vi "WT330.vi"(7 "simulazione":bool, 8 "error in (no error)":errorcluster, 11 "Queue Name":string="WT330_Q") -> (0 "error out":errorcluster, 2 "Stopped":bool)   [LabVIEW 2019]
uses:
  TypeDef/MISURE WT.ctl
  TypeDef/DEVICE NAME.ctl
  <vilib>/Utility/file.llb/Read From Spreadsheet File (string).vi
  <instrlib>/Yokogawa WT300 Series/Public/Data/Read Measurement (Normal).vi
  Globals.vi
  Global_All_Data.vi
  <instrlib>/Yokogawa WT300 Series/Yokogawa WT300 Series.lvlib
  <instrlib>/Yokogawa WT200 Series/Yokogawa WT200 Series.lvlib
panel:
  out "error out 5":errorcluster
  out "error out 4":errorcluster
  in  "DIRETTO WT":bool
  out "error out 3":errorcluster
  in  "CT Ratio (1.000)":dbl=0.2 format="%#_13g"
  in  "write buffer":string=":INP:CURR:AUTO OFF;:INP:CURR:RANG EXT,1.0;"
  in  "LEM GENERICO":bool
  in  "Number of Item (15)":i32=39
  in  "rms mode":bool
  in  "dc mode":bool
  in  "IRMS 3":dbl
  out "error out 2":errorcluster
  in  "LEM 1000":bool
  in  "LEM 300":bool
  out "Numeric":i32
  in  "Measurement 2":dbl[](array[numeric])=[400.0, 25.0, 2409.0, 3031.0, 7.7, 0.8, 120.0, 50.0, 50.0, -1.0, 400.0, 25.0, 2409.0, 3031.0, 7.7, 0.8, 120.0, 50.0, 50.0, -1.0, 400.0, 25.0, 3030.0, 2400.0, 6.0, 0.8, 120.0, 50.0, 50.0, -1.0, 400.0, 25.0, 10104.0, 8009.0, 23.0, 0.8, 120.0, 50.0, 50.0]
  out "MISURE WT":T1
  out "WT330 Configuration":string[][](array[string])
  out "Function":string[](array[string])=["U,1\n", "I,1\n", "P,1\n", "S,1\n", "Q,1\n", "LAMB,1\n", "PHI,1\n", "FU,1\n", "FI,1\n", "NONE\n", "U,2\n", "I,2\n", "P,2\n", "S,2\n", "Q,2\n", "LAMB,2\n", "PHI,2\n", "FU,2\n", "FI,2\n", "NONE\n", "U,3\n", "I,3\n", "P,3\n", "S,3\n", "Q,3\n", "LAMB,3\n", "PHI,3\n", "FU,3\n", "FI,3\n", "NONE\n", "U,SIGM\n", "I,SIGM\n", "P,SIGM\n", "S,SIGM\n", "Q,SIGM\n", "LAMB,SIGM\n", "PHI,SIGM\n", "FU,SIGM\n", "FI,SIGM\n"]
  out "Measurement":dbl[](array[numeric])
  out "VISA resource name":refnum<visa-resource-name>
  out "STATO":string
  out "LOOP TIME (ms)":u32
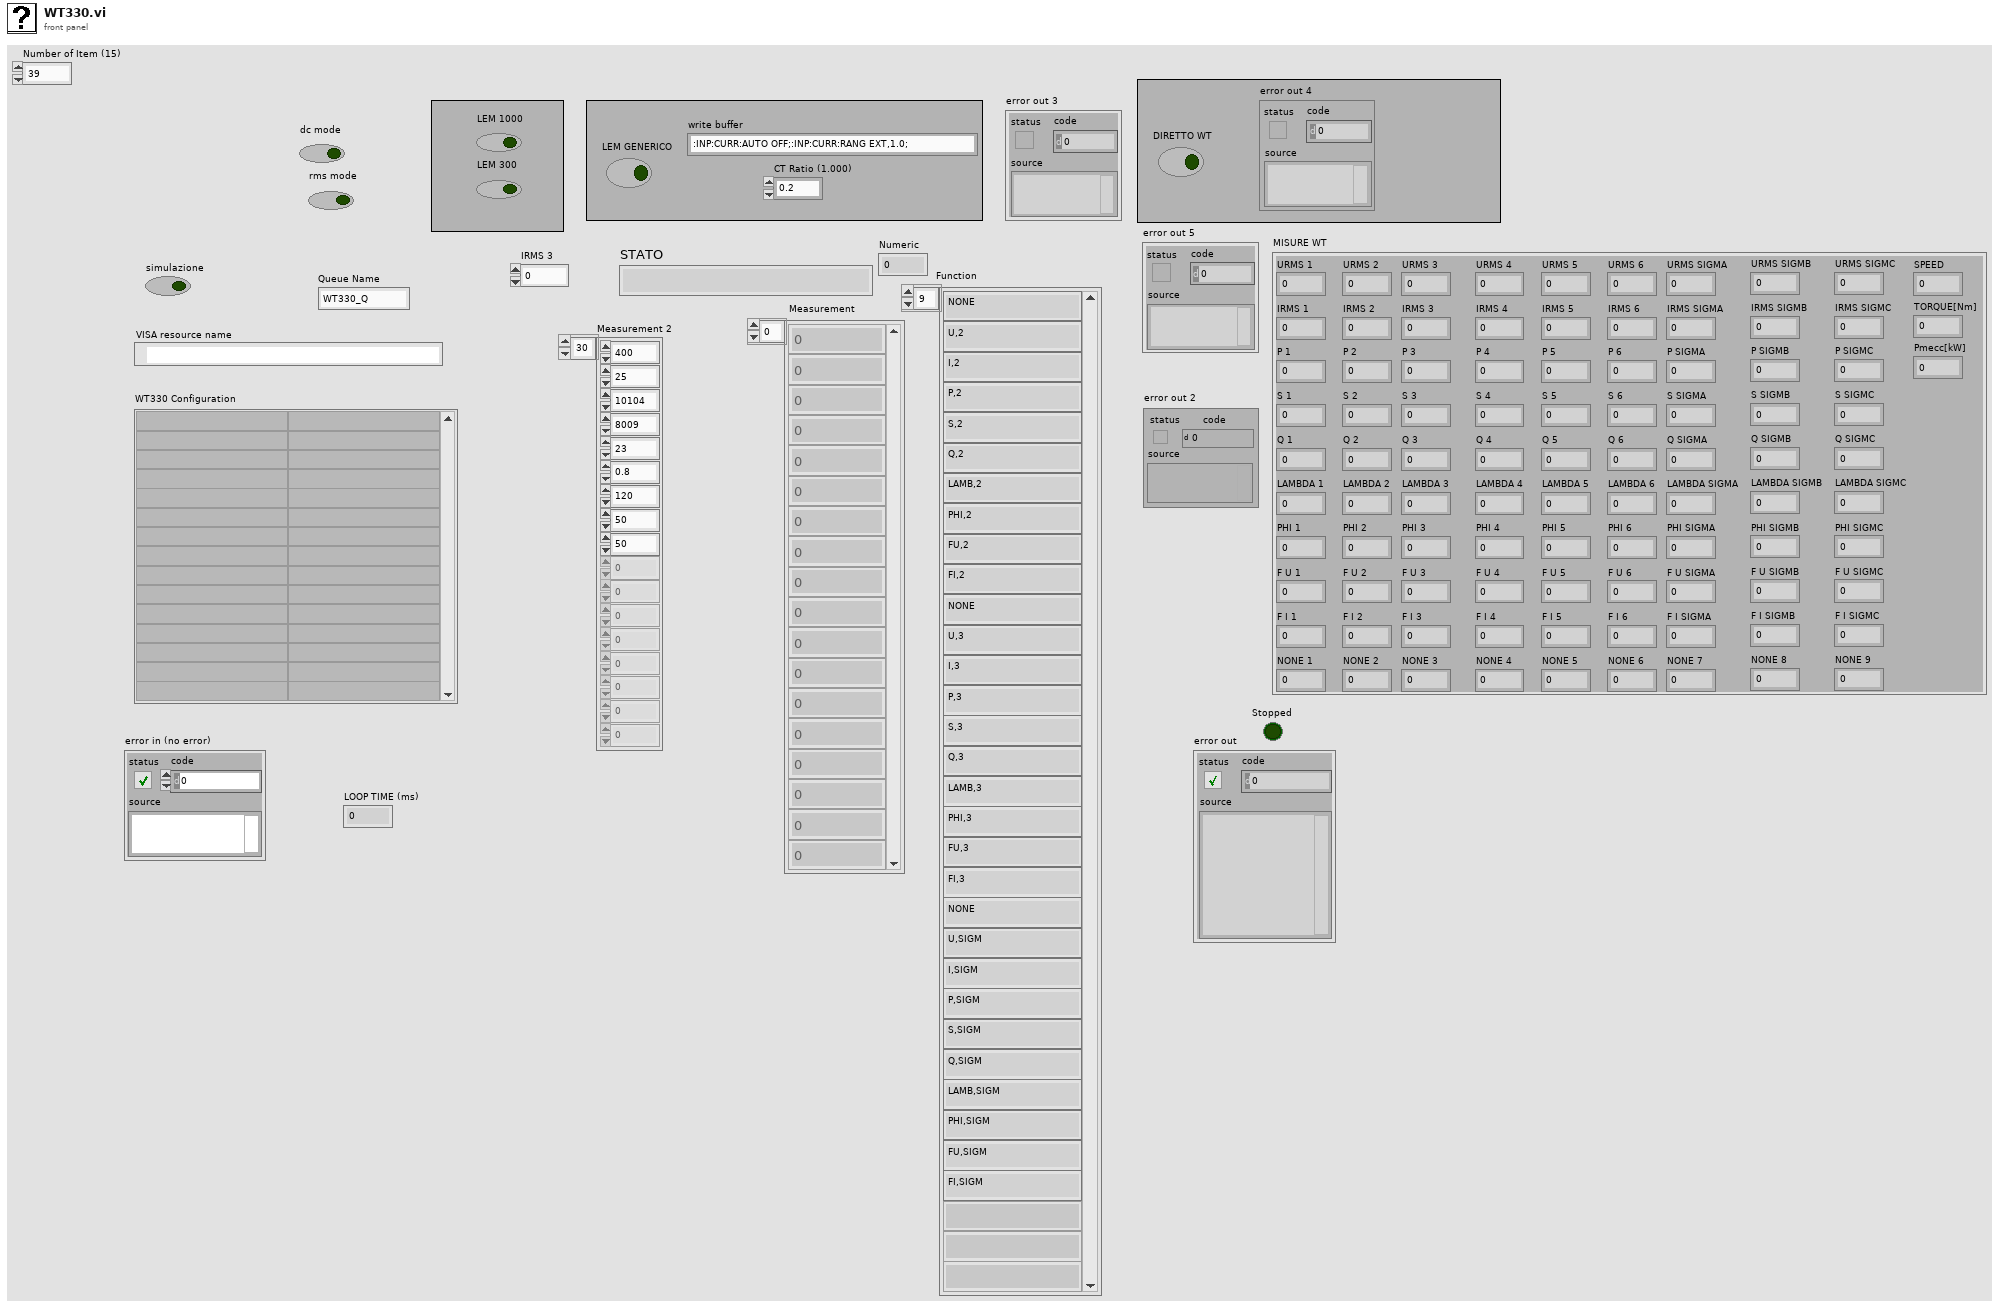
[diagram p1: front panel]
types:
  T1 = typedef "MISURE WT.ctl" = cluster{"URMS 1":dbl, "IRMS 1":dbl, "P 1":dbl, "S 1":dbl, "Q 1":dbl, "LAMBDA 1":dbl, "PHI 1":dbl, "F U 1":dbl, "F I 1":dbl, "NONE 1":dbl, "URMS 2":dbl, "IRMS 2":dbl, "P 2":dbl, "S 2":dbl, "Q 2":dbl, "LAMBDA 2":dbl, "PHI 2":dbl, "F U 2":dbl, "F I 2":dbl, "NONE 2":dbl, "URMS 3":dbl, "IRMS 3":dbl, "P 3":dbl, "S 3":dbl, "Q 3":dbl, "LAMBDA 3":dbl, "PHI 3":dbl, "F U 3":dbl, "F I 3":dbl, "NONE 3":dbl, "URMS 4":dbl, "IRMS 4":dbl, "P 4":dbl, "S 4":dbl, "Q 4":dbl, "LAMBDA 4":dbl, "PHI 4":dbl, "F U 4":dbl, "F I 4":dbl, "NONE 4":dbl, "URMS 5":dbl, "IRMS 5":dbl, "P 5":dbl, "S 5":dbl, "Q 5":dbl, "LAMBDA 5":dbl, "PHI 5":dbl, "F U 5":dbl, "F I 5":dbl, "NONE 5":dbl, "URMS 6":dbl, "IRMS 6":dbl, "P 6":dbl, "S 6":dbl, "Q 6":dbl, "LAMBDA 6":dbl, "PHI 6":dbl, "F U 6":dbl, "F I 6":dbl, "NONE 6":dbl, "URMS SIGMA":dbl, "IRMS SIGMA":dbl, "P SIGMA":dbl, "S SIGMA":dbl, "Q SIGMA":dbl, "LAMBDA SIGMA":dbl, "PHI SIGMA":dbl, "F U SIGMA":dbl, "F I SIGMA":dbl, "NONE 7":dbl, "URMS SIGMB":dbl, "IRMS SIGMB":dbl, "P SIGMB":dbl, "S SIGMB":dbl, "Q SIGMB":dbl, "LAMBDA SIGMB":dbl, "PHI SIGMB":dbl, "F U SIGMB":dbl, "F I SIGMB":dbl, "NONE 8":dbl, "URMS SIGMC":dbl, "IRMS SIGMC":dbl, "P SIGMC":dbl, "S SIGMC":dbl, "Q SIGMC":dbl, "LAMBDA SIGMC":dbl, "PHI SIGMC":dbl, "F U SIGMC":dbl, "F I SIGMC":dbl, "NONE 9":dbl, "SPEED":dbl, "TORQUE[Nm]":dbl, "Pmecc[kW]":dbl}
  T2 = typedef "DEVICE NAME.ctl" = enum16{"WATTMETRO", "APLUS", "PLC BANCO 1", "PLC RACK", "PLC BANCO 2", "PS", "NI cDAQ", "RESISTOMAT"}
  T3 = cluster{"Array of elements":cluster{"String":string, "variant":variant}[], "Single element":cluster{"String":string, "variant":variant}, "enque at\nopposite end (F)":bool, "no replications (F)":bool}
  T4 = cluster{"Measure Value[0]":dbl, "Measure Value[1]":dbl, "Measure Value[2]":dbl, "Measure Value[3]":dbl, "Measure Value[4]":dbl, "Measure Value[5]":dbl, "Measure Value[6]":dbl, "Measure Value[7]":dbl, "Measure Value[8]":dbl, "Measure Value[9]":dbl, "Measure Value[10]":dbl, "Measure Value[11]":dbl, "Measure Value[12]":dbl, "Measure Value[13]":dbl, "Measure Value[14]":dbl, "Measure Value[15]":dbl, "Measure Value[16]":dbl, "Measure Value[17]":dbl, "Measure Value[18]":dbl, "Measure Value[19]":dbl, "Measure Value[20]":dbl, "Measure Value[21]":dbl, "Measure Value[22]":dbl, "Measure Value[23]":dbl, "Measure Value[24]":dbl, "Measure Value[25]":dbl, "Measure Value[26]":dbl, "Measure Value[27]":dbl, "Measure Value[28]":dbl, "Measure Value[29]":dbl, "Measure Value[30]":dbl, "Measure Value[31]":dbl, "Measure Value[32]":dbl, "Measure Value[33]":dbl, "Measure Value[34]":dbl, "Measure Value[35]":dbl, "Measure Value[36]":dbl, "Measure Value[37]":dbl, "Measure Value[38]":dbl, "Measure Value[39]":dbl, "Measure Value[40]":dbl, "Measure Value[41]":dbl, "Measure Value[42]":dbl, "Measure Value[43]":dbl, "Measure Value[44]":dbl, "Measure Value[45]":dbl, "Measure Value[46]":dbl, "Measure Value[47]":dbl, "Measure Value[48]":dbl, "Measure Value[49]":dbl, "Measure Value[50]":dbl, "Measure Value[51]":dbl, "Measure Value[52]":dbl, "Measure Value[53]":dbl, "Measure Value[54]":dbl, "Measure Value[55]":dbl, "Measure Value[56]":dbl, "Measure Value[57]":dbl, "Measure Value[58]":dbl, "Measure Value[59]":dbl, "Measure Value[60]":dbl, "Measure Value[61]":dbl, "Measure Value[62]":dbl, "Measure Value[63]":dbl, "Measure Value[64]":dbl, "Measure Value[65]":dbl, "Measure Value[66]":dbl, "Measure Value[67]":dbl, "Measure Value[68]":dbl, "Measure Value[69]":dbl, "Measure Value[70]":dbl, "Measure Value[71]":dbl, "Measure Value[72]":dbl, "Measure Value[73]":dbl, "Measure Value[74]":dbl, "Measure Value[75]":dbl, "Measure Value[76]":dbl, "Measure Value[77]":dbl, "Measure Value[78]":dbl, "Measure Value[79]":dbl, "Measure Value[80]":dbl, "Measure Value[81]":dbl, "Measure Value[82]":dbl, "Measure Value[83]":dbl, "Measure Value[84]":dbl, "Measure Value[85]":dbl, "Measure Value[86]":dbl, "Measure Value[87]":dbl, "Measure Value[88]":dbl, "Measure Value[89]":dbl, "Measure Value[90]":dbl, "Measure Value[91]":dbl, "Measure Value[92]":dbl}
  T5 = typedef "Cluster MISURE.ctl" = cluster{"MISURE NM":T6, "MISURE ALL":T7}
  T6 = typedef "MISURE NM.ctl" = cluster{"Banco":string, "Anno":string, "Numero":string, "Ntabella":string, "Misura":string, "Tipo Prova":string, "ProgressivoAcq":string, "Descrizione":string, "Data_ora":string, "t. acq [h:m:s]":string, "t. acq [min]":string, "t. acq [s]":string, "n [rpm]":string, "f [Hz]":string, "U1[V]":string, "U2 [V]":string, "U3 [V]":string, "U123_media [V]":string, "I1[A]":string, "I2[A]":string, "I3[A]":string, "I123_media [A]*I":string, "I_123_sbil [%]":string, "Ulin[V]":string, "Uc [V]":string, "Uaux [V]":string, "Ilin[A]*I":string, "Imar[A]":string, "Iaux[A]":string, "Uarm[V]":string, "Uecc[V]":string, "Iarm[A]*I":string, "Iecc[A]":string, "pf":string, "P1 [W]":string, "P1 [kW]":string, "Q [VAR]":string, "Q [kVAR]":string, "S [VA]":string, "S [kVA]":string, "P1arm[W]":string, "P1ecc[W]":string, "Parm[kW]":string, "P1ecc[kW]":string, "Cond[uF]":string, "P1_linea_6fili[W]":string, "P1_linea_6fili[kW]":string, "eta_gr_6fili [%]":string, "eta_inverter_6fili [%]":string, "pf_linea_6fili":string, "U4 [V]":string, "U5 [V]":string, "U6 [V]":string, "U456_media [V]":string, "I4 [A]":string, "I5 [A]":string, "I6 [A]":string, "I456_media [A]":string, "C [Nm]*C":string, "Cric [Nm]":string, "Cric\\Cnom":string, "Iric[A]":string, "Iric\\Inom":string, "P2_mecc [W]":string, "P2_mecc [kW]":string, "eta motore [%]":string, "Scorr[%]":string, "Tamb[°C]":string, "R1[ohm]":string, "R2[ohm]":string, "R3[ohm]":string, "Rmedia[ohm]":string, "DT_R1[°C]":string, "DT_R2[°C]":string, "DT_R3[°C]":string, "DT_media[°C]":string, "R_marcia[ohm]":string, "R_aux[ohm]":string, "DT_marcia[°C]":string, "DT_aux[°C]":string, "R_Arm[ohm]":string, "R_Ecc[ohm]":string, "DT_Arm[°C]":string, "DT_Ecc[°C]":string, "TambFreddo[°C]":string, "R1_freddo[ohm]":string, "R2_freddo[ohm]":string, "R3_freddo[ohm]":string, "Rmedia_freddo[ohm]":string, "R_Marcia_freddo[ohm]":string, "R_Aux_freddo[ohm]":string, "R_Arm_freddo[ohm]":string, "R_Ecc_freddo[ohm]":string, "TC1 [°C]":string, "TC2 [°C]":string, "TC3 [°C]":string, "TC4 [°C]":string, "TC5 [°C]":string, "TC6 [°C]":string, "TC7 [°C]":string, "TC8 [°C]":string, "PT1000_1[°C]":string, "PT1000_2[°C]":string, "PT1000_3[°C]":string, "Vdc eccitatrice[V]":string, "Idc eccitatrice[A]":string, "Vdc rotore[V]":string, "Idc rotore[A]":string, "Vac rotore[V]":string, "Iac rotore[V]":string, "V dinamo[V]":string, "Portata Q":string, "Pressione H":string, "U1'[V]":string, "U2'[V]":string, "U3'[V]":string, "I1'[A]":string, "I2'[A]":string, "I3'[A]":string, "U''R-N":string, "U''S-N":string, "U'' T-N":string, "U''R-S":string, "U''R-T":string, "U''S-T":string, "I1''[A]":string, "I2''[A]":string, "I3''[A]":string, "F''[Hz]":string, "P''[kW]":string, "CosFi''":string, "PT1000_4[°C]":string, "Scorta 3":string}
  T7 = typedef "Cluster misure ALL.ctl" = cluster{"Cluster READ NI":T8, "MISURE WT":T1, "Resistenze Resistomat":T11, "INTERFACCIA":T12, "FREDDO resistomat":cluster{"Res Ch1":dbl, "Res Ch2":dbl, "tAMB":dbl, "Res Ch3":dbl}, "STATO PLC 1":T17, "Res Ch2":dbl, "Res Ch2 2":dbl, "FREDDO res meter":cluster{"Res Ch1":dbl, "Res Ch2":dbl, "tAMB":dbl, "Res Ch3":dbl}, "Resistenze Res Meter":T11, "READ SINUS PENTA":T21, "STATO PLC 2":T22, "STATO PLC 3":T26, "DCREG":T30}
  T8 = typedef "Cluster NI.ctl" = cluster{"AI (0-10V)":cluster{"AI 0":dbl, "AI 1":dbl, "AI 2":dbl, "AI 3":dbl, "AI 4":dbl, "AI 5":dbl, "AI 6":dbl, "AI 7":dbl, "AI 8":dbl, "AI 9":dbl, "AI 10":dbl, "AI 11":dbl, "AI 12":dbl, "AI 13":dbl, "AI 14":dbl, "AI 15":dbl, "AI 16":dbl, "AI 17":dbl, "AI 18":dbl, "AI 19":dbl, "AI 20":dbl, "AI 21":dbl, "AI 22":dbl, "AI 23":dbl, "AI 24":dbl, "AI 25":dbl, "AI 26":dbl, "AI 27":dbl, "AI 28":dbl, "AI 29":dbl, "AI 30":dbl, "AI 31":dbl}, "StatoAO_Cdaq[0-10V]":cluster{"AO 1":dbl, "AO 2":dbl, "AO 3":dbl, "AO 4":dbl}, "Contatori [rpm]":cluster{"RPM 1":dbl, "RPM 2":dbl}, "StatoAO_Cdaq [4-20mA]":T9, "StatoDO_Cdaq":T10, "DI":cluster{"Scorta 0":bool, "Scorta 1":bool, "Scorta 2":bool, "Scorta 3":bool, "Scorta 4":bool, "Scorta 5":bool, "Scorta 6":bool, "Scorta 7":bool, "Scorta 8":bool, "Scorta 9":bool, "Scorta 10":bool, "Scorta 11":bool, "Scorta 12":bool, "Scorta 13":bool, "Scorta 14":bool, "Scorta 15":bool, "Scorta 16":bool, "Scorta 17":bool, "Scorta 18":bool, "Scorta 19":bool, "Scorta 20":bool, "Scorta 21":bool, "Scorta 22":bool, "Scorta 23":bool, "Scorta 24":bool, "Scorta 25":bool, "Scorta 26":bool, "Scorta 27":bool, "Scorta 28":bool, "Scorta 29":bool, "Scorta 30":bool, "Scorta 31":bool}, "AI (4-20mA)":cluster{"AI 0":dbl, "AI 1":dbl, "AI 2":dbl, "AI 3":dbl, "AI 4":dbl, "AI 5":dbl, "AI 6":dbl, "AI 7":dbl, "AI 8":dbl, "AI 9":dbl, "AI 10":dbl, "AI 11":dbl, "AI 12":dbl, "AI 13":dbl, "AI 14":dbl, "AI 15":dbl}, "TC [°C]":cluster{"tc 1":dbl, "tc 2":dbl, "tc 3":dbl, "tc 4":dbl}}
  T9 = typedef "StatoAO_cdaq.ctl" = cluster{"Cdaq_AO [0-10V] 0":dbl, "Cdaq_AO [0-10V] 1":dbl, "Cdaq_AO [0-10V] 2":dbl, "Cdaq_AO [0-10V] 3":dbl, "Cdaq_AO [4-20mA] 0":dbl, "Cdaq_AO [4-20mA] 1":dbl, "Cdaq_AO [4-20mA] 2":dbl, "Cdaq_AO [4-20mA] 3":dbl, "Cdaq_AO [4-20mA] 4":dbl, "Cdaq_AO [4-20mA] 5":dbl, "Cdaq_AO [4-20mA] 6":dbl, "Cdaq_AO [4-20mA] 7":dbl}
  T10 = typedef "statoDO_Cdaq.ctl" = cluster{"Scorta 0":bool, "Scorta 1":bool, "Scorta 2":bool, "Scorta 3":bool, "Scorta 4":bool, "Scorta 5":bool, "Scorta 6":bool, "Scorta 7":bool, "Scorta 8":bool, "Scorta 9":bool, "Scorta 10":bool, "Scorta 11":bool, "Scorta 12":bool, "Scorta 13":bool, "Scorta 14":bool, "Scorta 15":bool, "Scorta 16":bool, "Scorta 17":bool, "Scorta 18":bool, "Scorta 19":bool, "Scorta 20":bool, "Scorta 21":bool, "Scorta 22":bool, "Scorta 23":bool, "Scorta 24":bool, "Scorta 25":bool, "Scorta 26":bool, "Scorta 27":bool, "Scorta 28":bool, "Scorta 29":bool, "Scorta 30":bool, "Scorta 31":bool}
  T11 = typedef "ClusterRes.ctl" = cluster{"Res Ch1":dbl, "Res Ch2":dbl, "Res Ch3":dbl, "Tamb":dbl}
  T12 = typedef "INTERFACCIA.ctl" = cluster{"AI":cluster{"Portate":T13[], "Pressioni":T13[], "Coppie[Nm]":T13[], "Valvole prop %":T13[], "RPM":T13[], "Livelli":T13[], "Temperature":T13[], "Riferimenti %":T13[], "TENSIONI":T13[], "CORRENTI":T13[]}, "DI (logici)":cluster{"Start da pulsantiera":bool, "Stop da pulsantiera":bool, "Reset da pulsantiera":bool, "Sistema OK":bool, "Collaudo abilitato":bool, "Potenza trifase abilitata":bool, "Potenza monofase abilitata":bool, "Potenza DC abilitata":bool, "Potenza DC ECC abilitata":bool, "Start alimentazione AC":bool, "Start alimentazione DC":bool, "Start DC eccitazione":bool, "Teleruttore WT abilitato":bool, "Teleruttore Resistomat abilitato":bool, "Teleruttore corto fasi":bool, "Ramo 1 resistomat":bool, "Ramo 2 resistomat":bool, "Ramo 3 resistomat":bool, "B1 Scelta linea elettrica 1":bool, "B1 Scelta linea elettrica 2":bool, "B1 Scelta linea elettrica 3":bool, "B1 Scelta linea elettrica 4":bool, "B1 Scelta linea elettrica 5":bool, "B2 Scelta linea elettrica 1":bool, "B2 Scelta linea elettrica 2":bool, "B2 Scelta linea elettrica 3":bool, "B2 Scelta linea elettrica 4":bool, "B2 Scelta linea elettrica 5":bool, "Rotore bloccato 1":bool, "Rotore bloccato 2":bool, "FRENO 1 abilitato":bool, "FRENO 1 run":bool, "FRENO 1 senso rotaz":bool, "FRENO 1 ctrl velocità":bool, "FRENO 2 abilitato":bool, "FRENO 2 run":bool, "FRENO 2 senso rotaz":bool, "FRENO 2 ctrl velocità":bool, "ALIM 1 abilitato":bool, "ALIM 1 run":bool, "ALIM 2 abilitato":bool, "ALIM 2 run":bool, "ALIM 3 abilitato":bool, "ALIM 3 run":bool, "FRENO 1 ctrl coppia":bool, "FRENO 2 ctrl coppia":bool, "FRENO 3 ctrl coppia":bool, "DI (logici) aggiuntivi impianto":cluster{"Solo freno abilitato":bool, "Carico resistivo abilitato":bool, "AFE+freno abilitato":bool, "Protezioni chiuse":bool, "Start potenza AFE":bool, "AFE in marcia":bool}, "Misura corrente diretta WT":bool, "Misura corrente sens ext":bool, "Sens ext abilitati":bool}, "AO non scalati":T15, "AO scalati":T15, "DO (logici)":T16}
  T13 = typedef "ClusterMisura_e_Unità_INPUT.ctl" = cluster{"Misura":dbl, "UM":T14, "Descrizione":string}
  T14 = typedef "UnitàMisura.ctl" = enum16{"V", "mA", "Bar", "RPM", "m3/s", "m3/min", "m3/h", "l/s", "l/min", "in3/min", "ft3/min", "gpm", "igpm", "igph", "%", "°C", "m", "Nm", "A"}
  T15 = typedef "Lista AO sistema.ctl" = cluster{"FRENO1 rif vel":dbl, "FRENO1 rif Coppia":dbl, "FRENO2 rif vel":dbl, "FRENO2 rif Coppia":dbl, "ALIM1 rif V":dbl, "ALIM1 rif F":dbl, "ALIM2 rif V":dbl, "ALIM2 rif F":dbl, "ALIM3 rif V":dbl, "ALIM3 rif F":dbl, "Fnom keb":dbl, "Rpm nom keb":dbl, "Pnom keb":dbl, "Inom keb":dbl, "Vnom keb":dbl, "Rpm max keb":dbl, "Tempo rampa keb":dbl, "Tipo Mot keb":dbl}
  T16 = typedef "DOinterfaccia.ctl" = cluster{"Scelta banco 1":bool, "Scelta banco 2":bool, "Scelta banco 3":bool, "FRENO 1 abilita":bool, "FRENO 1 start":bool, "FRENO 1 senso rotaz":bool, "FRENO 1 ctrl velocità":bool, "FRENO 2 abilita":bool, "FRENO 2 start":bool, "FRENO 2 senso rotaz":bool, "FRENO 2 ctrl velocità":bool, "ALIM 1 abilita":bool, "ALIM 1 start":bool, "ALIM 2 abilita":bool, "ALIM 2 start":bool, "ALIM 3 abilita":bool, "ALIM 3 start":bool, "Abilita linea trifase":bool, "Abilita linea monofase":bool, "Abilita linea dc":bool, "Abilita linea dc eccit":bool, "B1 Linea elettrica 1":bool, "B1 Linea elettrica 2":bool, "B1 Linea elettrica 3":bool, "B1 Linea elettrica 4":bool, "B1 Linea elettrica 5":bool, "B2 Linea elettrica 1":bool, "B2 Linea elettrica 2":bool, "B2 Linea elettrica 3":bool, "B2 Linea elettrica 4":bool, "B2 Linea elettrica 5":bool, "Start potenza AC":bool, "Stop pontenza AC":bool, "Start potenza DC":bool, "Stop potenza DC":bool, "Start potenza eccitaz":bool, "Stop potenza eccitaz":bool, "Reset allarmi":bool, "watchdog":bool, "Scala torsiometro B1":bool, "Controllo torsiom B1":bool, "Scala torsiometro B2":bool, "Controllo torsiom B2":bool, "Teleruttore WT abilita":bool, "Teleruttore Resistomat abilita":bool, "Teleruttore corto fasi":bool, "Ramo 1 resistomat":bool, "Ramo 2 resistomat":bool, "Ramo 3 resistomat":bool, "Collaudo in corso":bool, "Allarme presente":bool, "Enable Res Meter":bool, "Bypass Res Meter":bool, "2nd canale Res Meter":bool, "Scala 200/2000 res meter":bool, "Taratura res meter":bool, "FRENO 1 ctrl coppia":bool, "FRENO 2 ctrl coppia":bool, "FRENO 3 ctrl coppia":bool, "Aggiuntivi impianto":cluster{"Senso rotazione alim 1":bool, "Senso rotazione alim 2":bool}, "ALIM 1 stop":bool, "ALIM 2 stop":bool, "ALIM 3 stop":bool, "FRENO 1 stop":bool, "FRENO 2 stop":bool, "FRENO 3 stop":bool, "B1 configurazione freno B":bool, "B2 configurazione freno B":bool, "Abilita scrittura KEB":bool}
  T17 = typedef "STATO PLC 1.ctl" = cluster{"USCITE PLC":T18, "Stato DI_PLC":cluster{"Sistema OK":bool, "Rotore bloccato":bool, "Scorta 1":bool, "Prova diretto inverter":bool, "Prova con filtro LC":bool, "Teleruttore WT abilitato":bool, "Alim sinus penta abilitato":bool, "Alim sinus penta in marcia":bool, "Freno abilitato":bool, "Freno in marcia":bool, "Senso rotazione freno":bool, "Potenza abilitata":bool, "Scorta 3":bool, "Scorta 4":bool, "scorta 5":bool, "scorta 6":bool}, "AI plc":cluster{"Allarmi 1":dbl, "Allarmi 2":dbl, "Scorta 1":dbl, "Scorta 2":dbl, "RPM mot prova":dbl, "I mot prova":dbl, "RPM freno":dbl, "I freno":dbl, "Scorta 3":dbl, "Scorta 4":dbl}}
  T18 = typedef "Uscite PLC 1.ctl" = cluster{"AO (real) 2":cluster{"SCORTA 1":dbl, "SCORTA 2":dbl, "SCORTA 3":dbl, "SCORTA 4":dbl, "SCORTA 5":dbl, "SCORTA 6":dbl, "SCORTA 7":dbl, "SCORTA 8":dbl}, "statoAO_PLC out":T19, "DO (bit)":T20}
  T19 = typedef "statoAO_plc_1.ctl" = cluster{"Rif Lim coppia freno [%]":dbl, "Rif rpm freno [%]":dbl, "Rif coppia freno [%]":dbl, "Rif V alimentatore [%]":dbl, "Rif F alimentatore [%]":dbl}
  T20 = typedef "StatoDO_PLC_1.ctl" = cluster{"Scelta banco 1":bool, "Set dati motore freno 2":bool, "Diretto inverter":bool, "Filtro LC":bool, "Marcia ALIM (1s)":bool, "Marcia FRENO (1s)":bool, "Stop AFE (1s)":bool, "Stop freno (1s)":bool, "Reset allarmi":bool, "Watchdog":bool, "Senso rotazione":bool, "Abilita collaudo (1s)":bool, "Disabilita collaudo (1s)":bool, "Abilitazione ALIM":bool, "Abilitazione FRENO":bool, "Teleruttore WT":bool, "Senso rot motore prova":bool, "Scorta 7":bool, "Scorta 8":bool, "Scorta 9":bool, "Scorta 10":bool, "Scorta 11":bool, "Scorta 12":bool, "Scorta 13":bool}
  T21 = typedef "Parametri inverter letti.ctl" = cluster{"Menù Misure motore (M000-M030)":cluster{"Rif vel a regime (int)":u16, "Rif vel a regime (dec)":u16, "Rif vel dopo rampe (int)":u16, "Rif vel dopo rampe (dec)":u16, "RPM motore (int)":u16, "RPM motore (dec)":u16, "FREQout inverter":u16, "Rif coppia a regime(Nm)":u16, "Richiesta di coppia (Nm)":u16, "Coppia generata dal motore(Nm)":u16, "Rif coppia a regime(%)":u16, "Richiesta di coppia (%)":u16, "Coppia generata dal motore(%)":u16, "Coppia max richiesta prima delle rampe(Nm)":u16, "Coppia max richiesta dopo le rampe(Nm)":u16, "Limite di velocità prima delle rampe":u16, "Limite di velocità dopo le rampe":u16, "Coppia max richiesta prima delle rampe(%)":u16, "Coppia max richiesta dopo le rampe(%)":u16, "Rif di flusso":u16, "Corrente di uscita":u16, "Capacità termica del motore":u16, "Tensione di uscita":u16, "Potenza di uscita":u16, "Energia consumata (LSword)":u16, "Energia consumata (MSword)":u16, "Tensione bus DC":u16, "Tensione di rete":u16}, "Menù regolatore PID (M018-M024)":cluster{"Rif PID a regime(%)":u16, "Rif pid dopo rampe(%)":u16, "Retroazione del pid(%)":u16, "Errore del pid(%)":u16, "uscita del pid(%)":u16, "Rif del pid dopo le rampe":u16, "Retroazione del pid":u16}, "Menù ingressi digitali (M031-M036)":cluster{"Ingressi digitali ritardati":u16, "Ingressi digitali istantanei":u16, "Moresettiera comando loc":u16, "Morsett comando da seriale":u16, "Morsett comando bus di campo":u16, "Ing dig ausiliari da morsettiera":u16, "Ing dig ausiliari da seriale":u16}, "Menù riferimenti (M037-M051)":cluster{"Rif analog est REF":u16, "Rif analog est AIN1":u16, "Rif analog est AIN2":u16, "Rif analog est XAIN4":u16, "Rif analog est XAIN5":u16, "Rif velocità da seriale(int)":u16, "Rif velocità bus di campo(int)":u16, "Rif coppia da seriale":u16, "Rif coppia bus di campo":u16, "Rif del PID da seriale":u16, "Rif del PID da bus di campo":u16, "Retroazione del PID da seriale":u16, "Retroazione del PIDda bus di campo":u16, "Rif da encoder":u16, "Rif in frequenza":u16, "Rif velocità da seriale(dec)":u16, "Rif velocità bus di campo(dec)":u16}, "Menù rampe (P009-P033)":cluster{"Tempo di dec rampa di vel 1":u16, "Tempo di acc rampa di vel 2":u16, "Tempo di dec rampa di vel 2":u16, "Tempo di acc rampa di vel 1":u16, "Unità di mis tempi rampe vel 1/2":u16, "Tempo di acc rampa di vel 3":u16, "Tempo di dec rampa di vel 3":u16, "Tempo di acc rampa di vel 4":u16, "Tempo di dec rampa di vel 4":u16, "Unità di mis tempi rampe vel 3/4":u16, "Selettore arrottondam rampe":u16, "Tempo di arrotond iniz rampa acc":u16, "Tempo di arrotond finale rampa acc":u16, "Tempo di arrotond iniz rampa dec":u16, "Tempo di rampa di salita rif coppia":u16, "Tempo di rampa di discesa rif coppia":u16, "Unità di misura rampa coppia":u16, "Tempo rampa acc marcia jog":u16, "Tempo rampa dec marcia jog":u16, "Reset acc ai cambi pendenza":u16, "rampa di acc in fire mode":u16, "rampa di dec in fire mode":u16, "Tempo di arrotond finale rampa dec":u16}, "Menù controllo motore(C008-C128)":cluster{"Numero motori configurati":u16, "Tipo algoritmo di controllo Mot1":u16, "Tipo rif Mot1":u16, "Tensione nominale rete":u16, "Retroaz di vel da encoder Mot1":u16, "Tipo curva V/f Mot1":u16, "Rotazione delle fasi Mot1":u16, "Freq nominale del motore Mot1":u16, "RPM nominali del motore Mot1":u16, "Potenza nominale del motore Mot1":u16, "Corrente nominale del motore Mot1":u16, "Tensione nominale del motore mot1":u16, "Potenza a vuoto del motore Mot1":u16, "Corrente a vuoto del motore Mot1":u16, "Resistenza statorica del motore Mot1":u16, "Induttanza di dispersione Mot1":u16, "Induttanza mutua motore":u16, "Costante di tempo rotorica":u16, "Costante di tempo filtro pb":u16, "Velocità minima motore":u16, "Velocità massima motore":u16}, "Menù configurazione PID":cluster{"Selezione riferimento n.1":u16, "Selezione retroazione n.1":u16, "Modalità di fuzionamento PID":u16, "Termine derivativo calcolato su err o mis":u16, "Proporz moltiplica deriv e integrale":u16, "Azione del PID":u16}, "ID":dbl, "Menù uscite digitali":cluster{"MDO4 Inverter pronto":u16}, "Fcarrier":cluster{"Fcarrier Min (Hz)":u16, "Fcarrier Max (Hz)":u16}, "stato inverter M089":dbl, "Riferimenti":cluster{"Rif tensione":u16, "Rif velocità":u16}, "Comunicazione":bool, "Modalità stop":dbl}
  T22 = typedef "STATO PLC 2.ctl" = cluster{"USCITE PLC":T23, "Stato DI_PLC":cluster{"Sistema ok":bool, "Relè Resistomat abilitato":bool, "scorta d":bool, "scorta c":bool, "scorta b":bool, "scorta a":bool, "scorta 1":bool, "scorta 2":bool, "scorta 3":bool, "scorta 4":bool, "Scorta 5":bool, "Scorta 6":bool, "Scorta 7":bool, "Scorta 8":bool, "Scorta 9":bool, "Scorta 10":bool}, "AI plc":cluster{"Allarmi 1":dbl, "Allarmi 2":dbl, "TC 1":dbl, "TC 2":dbl, "TC 3":dbl, "TC 4":dbl, "TC 5":dbl, "TC 6":dbl, "TC 7":dbl, "TC 8":dbl, "PT1000 1":dbl, "PT1000 2":dbl, "PT1000 3":dbl, "PT1000 4":dbl}}
  T23 = typedef "Uscite PLC 2.ctl" = cluster{"AO (real) 2":cluster{"SCORTA 1":dbl, "SCORTA 2":dbl, "SCORTA 3":dbl, "SCORTA 4":dbl, "SCORTA 5":dbl, "SCORTA 6":dbl, "SCORTA 7":dbl, "SCORTA 8":dbl}, "statoAO_PLC out":T24, "DO (bit)":T25}
  T24 = typedef "statoAO_plc_2.ctl" = cluster{"Condensatori":dbl, "Scorta 1":dbl, "Scorta 2":dbl}
  T25 = typedef "StatoDO_PLC_2.ctl" = cluster{"Scala Torsiometro":bool, "Ctrl torsiometro":bool, "Relè misura resistomat":bool, "Watchdog":bool, "Misura res ramo 1":bool, "Misura res ramo 2":bool, "Misura res ramo 3":bool, "Scelta banco 2":bool, "Reset allarmi":bool, "Reset centraline":bool, "Scorta 2":bool, "Scorta 3":bool, "Scorta 4":bool, "Scorta 5":bool, "Scorta 6":bool, "Scorta 7":bool}
  T26 = typedef "STATO PLC 3.ctl" = cluster{"USCITE PLC":T27, "Stato DI_PLC":cluster{"Sistema OK":bool, "Rotore bloccato":bool, "Filtro LC":bool, "Bypass Filtro LC":bool, "Scelta Trasformatore":bool, "Scelta Bypass trasformatore":bool, "Teleruttore wt abilitato":bool, "Alimentatore abilitato":bool, "Alimentatore in marcia":bool, "Freno abilitato":bool, "Freno in marcia":bool, "Freno senso di rotazione":bool, "Potenza abilitata":bool, "Alimentatore in allarme":bool, "Freno in allarme":bool, "Conferma dati KEB":bool, "Scorta 4":bool, "Scorta 5":bool, "Scorta 6":bool}, "AI plc":cluster{"Allarmi 1":dbl, "Allarmi 2":dbl, "RPM motore prova":dbl, "Corrente motore prova":dbl, "RPM freno":dbl, "Corrente freno":dbl, "Tipo motore keb":dbl, "I nom keb":dbl, "RPM nom keb":dbl, "V nom keb":dbl, "F nom keb":dbl, "T rampa keb":dbl, "scorta":dbl, "Scorta 2":dbl}}
  T27 = typedef "Uscite PLC 3.ctl" = cluster{"AO (real) 2":cluster{"SCORTA 1":dbl, "SCORTA 2":dbl, "SCORTA 3":dbl, "SCORTA 4":dbl, "SCORTA 5":dbl, "SCORTA 6":dbl, "SCORTA 7":dbl, "SCORTA 8":dbl}, "statoAO_PLC out":T28, "DO (bit)":T29}
  T28 = typedef "statoAO_plc_3.ctl" = cluster{"Rif limitazione coppia freno":dbl, "Rif velocità freno":dbl, "Rif coppia freno (predisp.)":dbl, "Rif velocità alimentatore":dbl, "Scorta":dbl, "Tipo Motore  keb":dbl, "I nom keb":dbl, "RPM nom keb":dbl, "V nom keb":dbl, "F nom keb":dbl, "t rampa keb":dbl, "scorta":dbl, "Scorta 2":dbl}
  T29 = typedef "StatoDO_PLC_3.ctl" = cluster{"Scelta banco 2":bool, "Abilita Scrittura Dati Keb":bool, "Filtro LC":bool, "Bypass filtro LC":bool, "Trasformatore":bool, "Bypass trasformatore":bool, "Marcia alimentatore (1s)":bool, "Marcia freno (1s)":bool, "Stop alimentatore (1s)":bool, "Stop freno (1s)":bool, "Reset allarmi":bool, "Watchdog":bool, "Freno senso di rotazione":bool, "Abilita pontenza (1s)":bool, "Disabilita potenza (1s)":bool, "Abilita alimentatore":bool, "Abilita freno":bool, "Teleruttore wt":bool, "Senso rot mot prova":bool, "Scorta":bool, "Scorta":bool, "Blocco elettroserrature":bool, "Scorta 6":bool, "Scorta 7":bool}
  T30 = typedef "Parametri DCREG letti.ctl" = cluster{"Parametri di misura":cluster{"M000":dbl, "M001":dbl, "M002":dbl, "M003":dbl, "M004":dbl, "M005":dbl, "M006":dbl, "M007":dbl, "M008":dbl, "M009":dbl, "M010":dbl, "M011":dbl, "M012":dbl, "M013":dbl, "M014":dbl, "M015":dbl, "M016":dbl, "M017":dbl, "M018":dbl, "M019":dbl, "M020":dbl, "M021":dbl, "M022":dbl, "M023":dbl, "M024":dbl, "M025":dbl, "M026":dbl, "M027":dbl, "M028":dbl, "M029":dbl, "M030":dbl, "M031":dbl}, "Parametri di programmazione":cluster{"P000":dbl, "P001":dbl, "P002":dbl, "P003":dbl, "P004":dbl, "P005":dbl, "P006":dbl, "P010":dbl, "P011":dbl, "P012":dbl, "P013":dbl, "P014":dbl, "P015":dbl, "P016":dbl, "P030":dbl, "P031":dbl, "P032":dbl, "P033":dbl, "P034":dbl, "P035":dbl, "P036":dbl, "P037":dbl, "P038":dbl, "P039":dbl, "P040":dbl, "P050":dbl, "P051":dbl, "P052":dbl, "P053":dbl, "P054":dbl, "P055":dbl, "P056":dbl, "P057":dbl, "P058":dbl, "P059":dbl, "P060":dbl, "P061":dbl, "P062":dbl, "P070":dbl, "P071":dbl, "P073":dbl, "P074":dbl, "P076":dbl, "P077":dbl, "P079":dbl, "P080":dbl, "P082":dbl, "P083":dbl, "P084":dbl, "P085":dbl, "P086":dbl, "P087":dbl, "P088":dbl, "P100":dbl, "P101":dbl, "P102":dbl, "P103":dbl, "P104":dbl, "P110":dbl, "P111":dbl, "P120":dbl, "P121":dbl, "P122":dbl, "P123":dbl, "P124":dbl, "P125":dbl, "P126":dbl, "P127":dbl, "P128":dbl, "P129":dbl, "P130":dbl, "P131":dbl, "P132":dbl, "P133":dbl, "P134":dbl, "P150":dbl, "P151":dbl, "P152":dbl, "P153":dbl, "P154":dbl, "P155":dbl, "P156":dbl, "P157":dbl, "P158":dbl, "P170":dbl, "P171":dbl, "P172":dbl, "P173":dbl, "P174":dbl, "P175":dbl, "P176":dbl, "P177":dbl, "P178":dbl, "P179":dbl, "P180":dbl, "P181":dbl, "P182":dbl, "P183":dbl, "P184":dbl, "P185":dbl, "P186":dbl, "P187":dbl, "P188":dbl, "P189":dbl, "P190":dbl, "P191":dbl, "P192":dbl, "P193":dbl, "P194":dbl, "P195":dbl, "P196":dbl, "P197":dbl, "P198":dbl, "P199":dbl, "P211":dbl, "P212":dbl, "P213":dbl, "P214":dbl, "P215":dbl, "P216":dbl, "P217":dbl, "P221":dbl, "P222":dbl, "P223":dbl, "P224":dbl, "P230":dbl, "P231":dbl, "P240":dbl, "P250":dbl, "P251":dbl}, "Parametri di configurazione":cluster{"C000":dbl, "C001":dbl, "C002":dbl, "C010":dbl, "C011":dbl, "C012":dbl, "C014":dbl, "C015":dbl, "C016":dbl, "C017":dbl, "C018":dbl, "C030":dbl, "C050":dbl, "C051":dbl, "C052":dbl, "C060":dbl, "C061":dbl, "C062":dbl, "C063":dbl, "C070":dbl, "C072":dbl, "C074":dbl, "C090":dbl, "C091":dbl, "C092":dbl, "C093":dbl, "C094":dbl, "C100":dbl, "C101":dbl, "C102":dbl, "C103":dbl, "C105":dbl, "C106":dbl, "C107":dbl, "C108":dbl, "C110":dbl, "C111":dbl, "C112":dbl, "C120":dbl, "C121":dbl, "C122":dbl, "C130":dbl, "C131":dbl, "C132":dbl, "C133":dbl, "C134":dbl, "C135":dbl, "C141":dbl, "C142":dbl, "C143":dbl, "C150":dbl, "C151":dbl, "C153":dbl, "C154":dbl, "C155":dbl, "C156":dbl, "C157":dbl, "C158":dbl, "C159":dbl, "C160":dbl, "C161":dbl, "C162":dbl, "C163":dbl, "C164":dbl, "C165":dbl, "C170":dbl}, "Codice allarme":dbl, "Comunicazione":bool}
  T31 = enum32{"Invalid", "Standard", "Closed", "Hidden", "Minimized", "Maximized"}
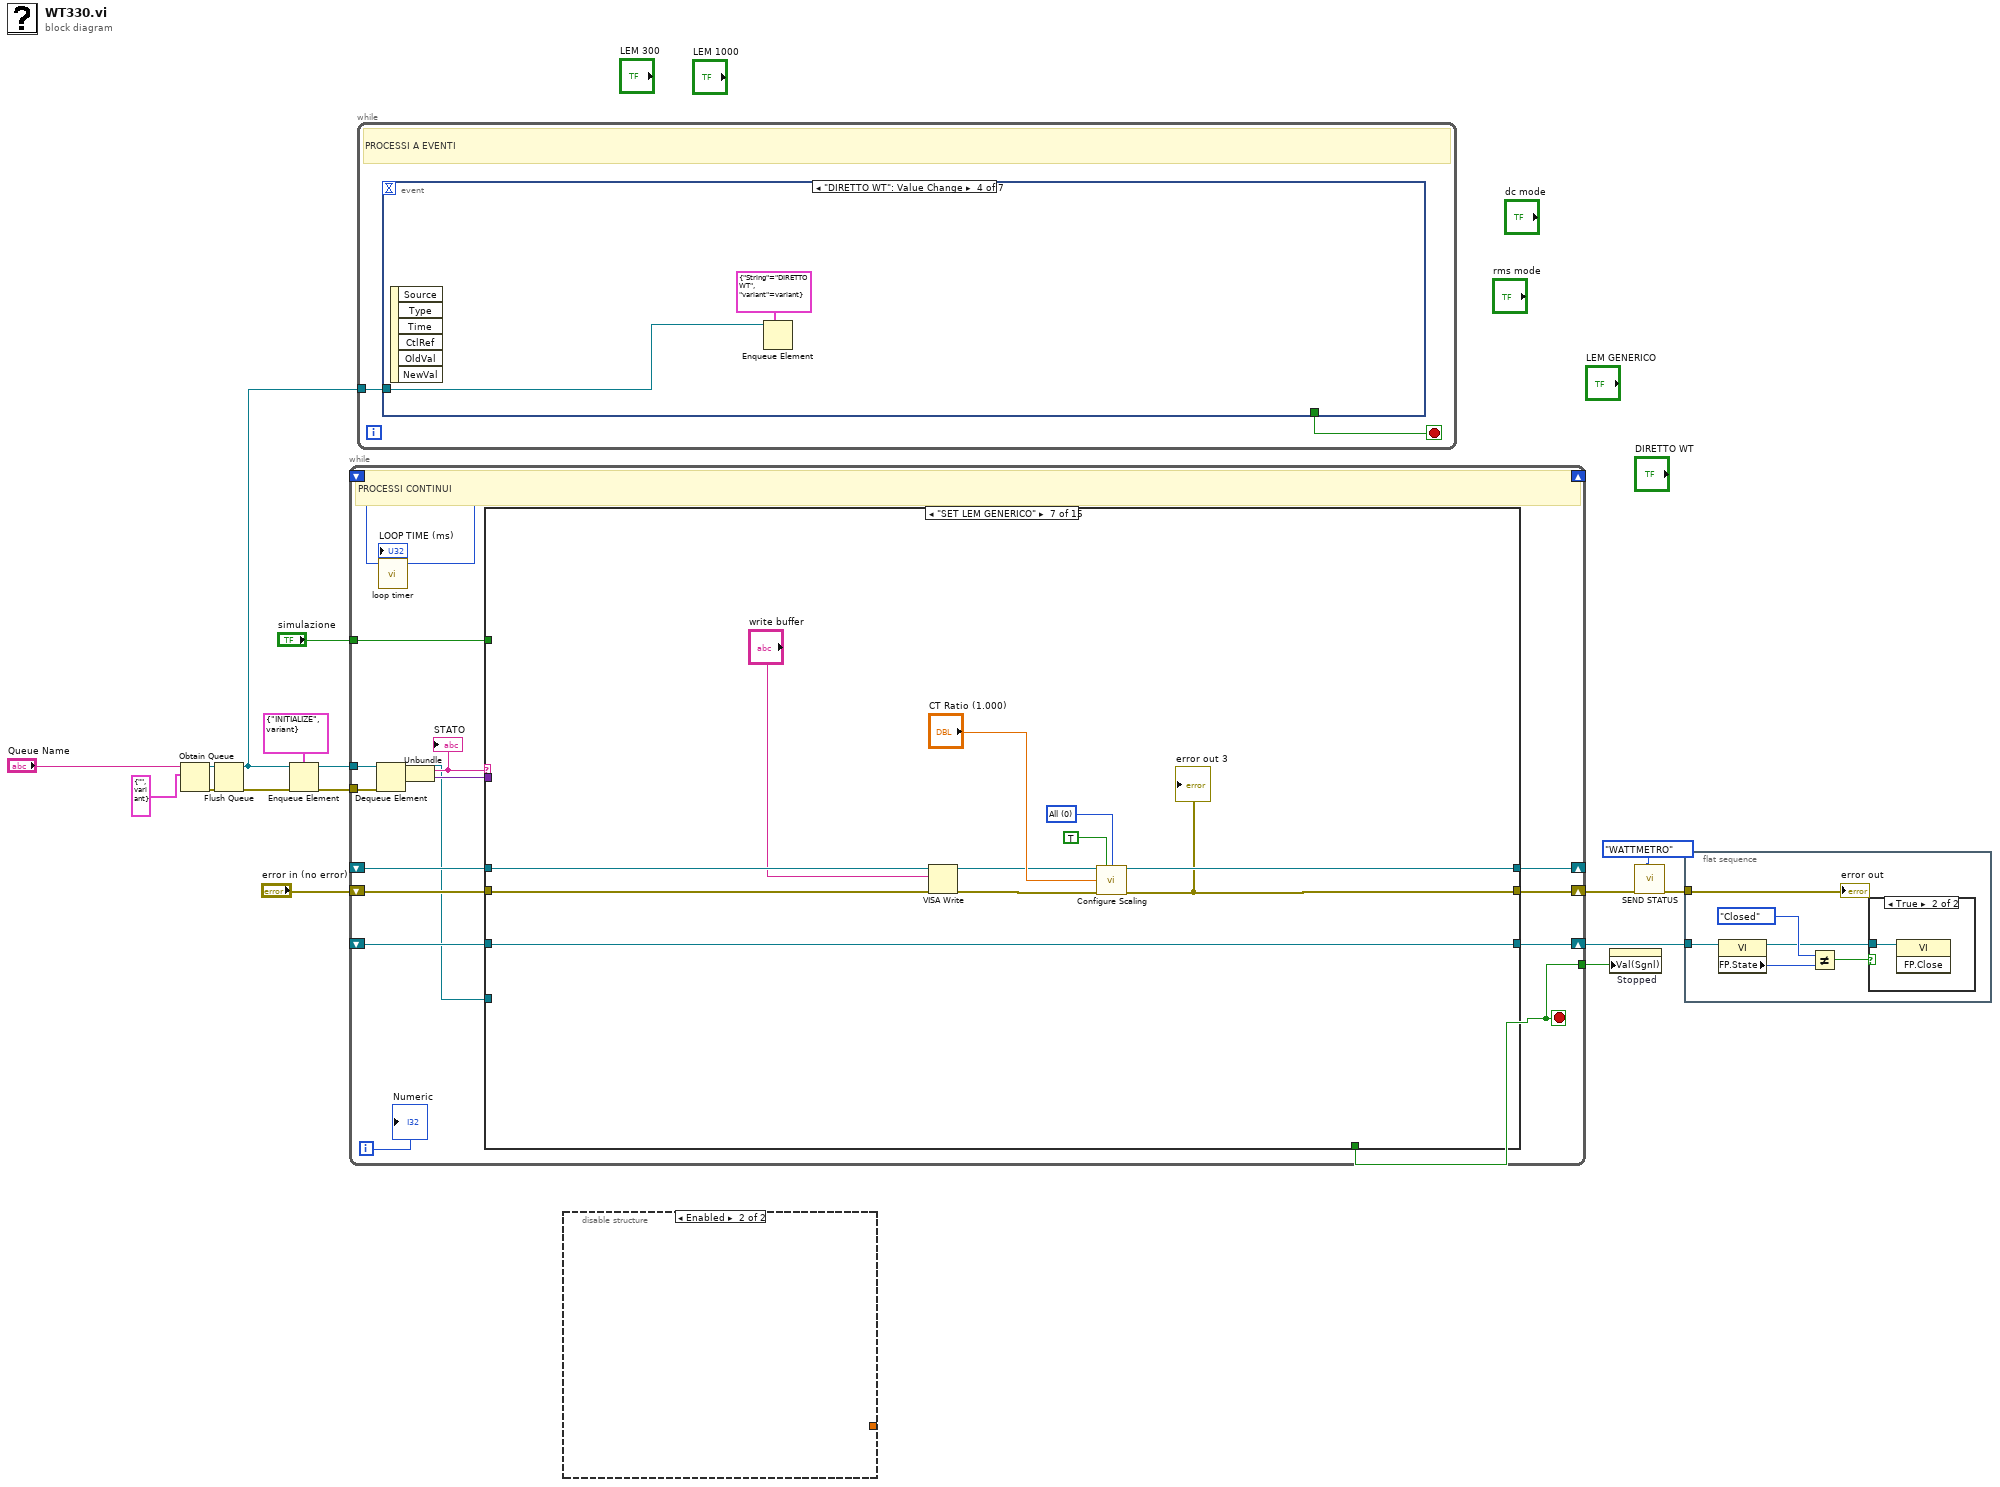
[diagram p0: block diagram]
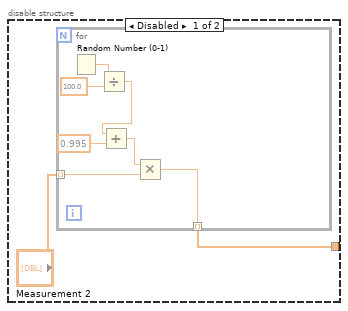
[diagram p2: hidden frame]
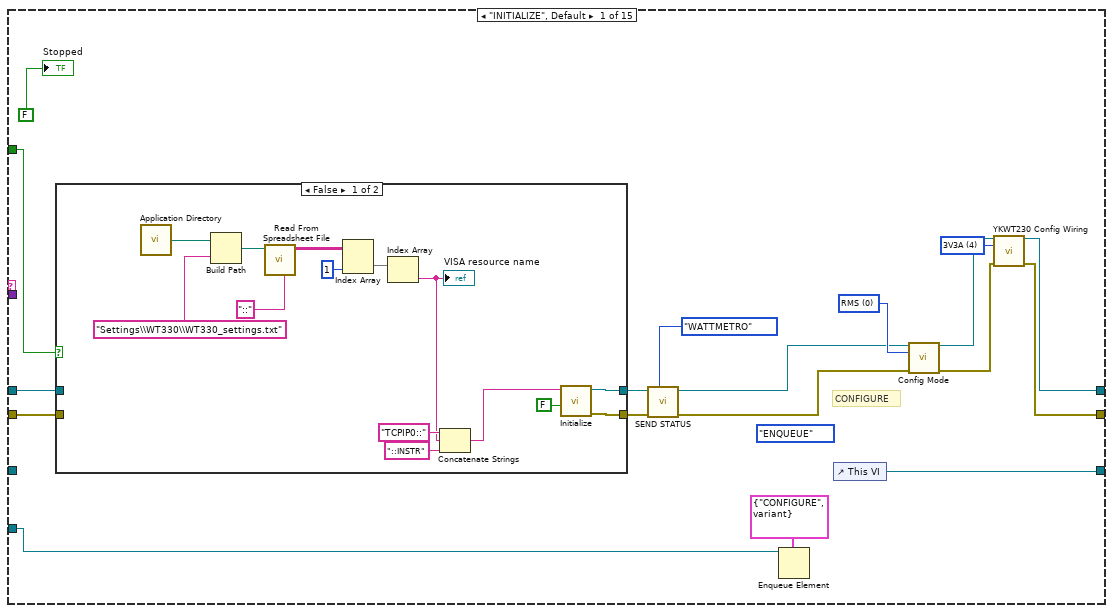
[diagram p4: hidden frame]
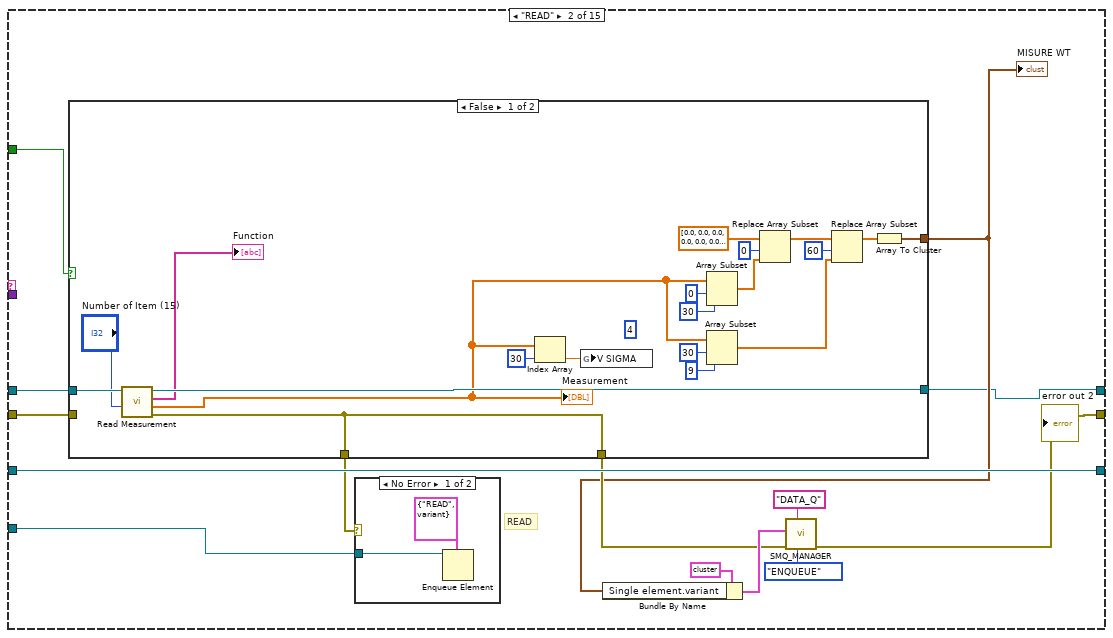
[diagram p6: hidden frame]
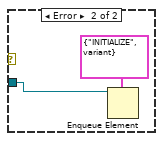
[diagram p7: hidden frame]
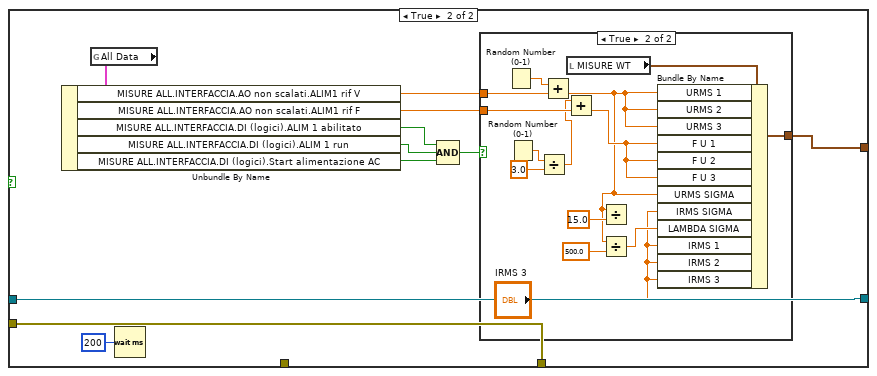
[diagram p8: hidden frame]
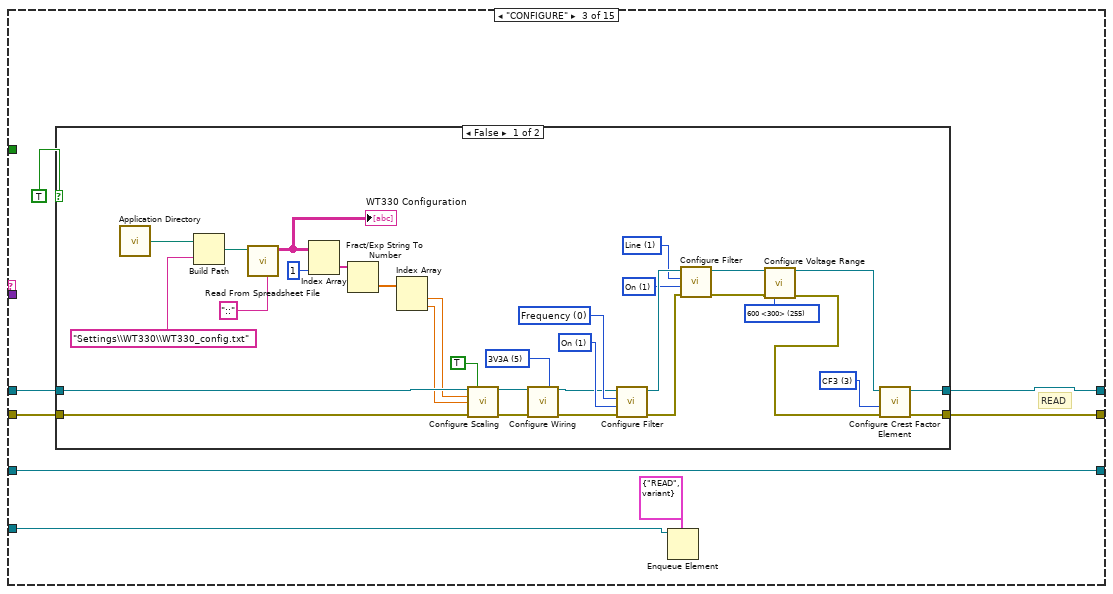
[diagram p10: hidden frame]
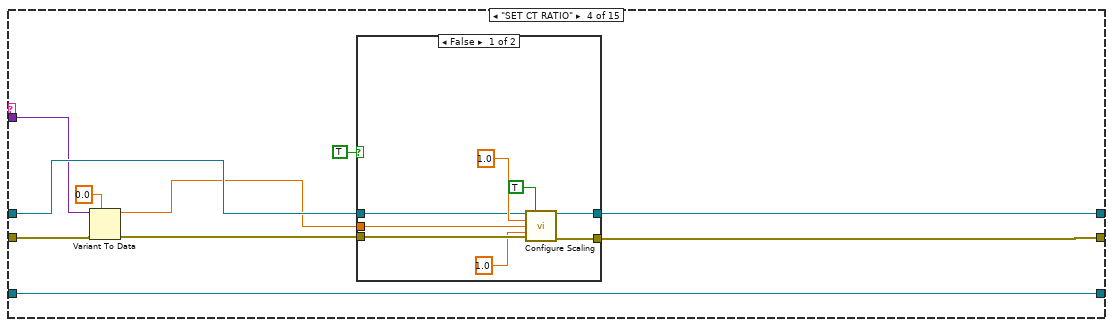
[diagram p12: hidden frame]
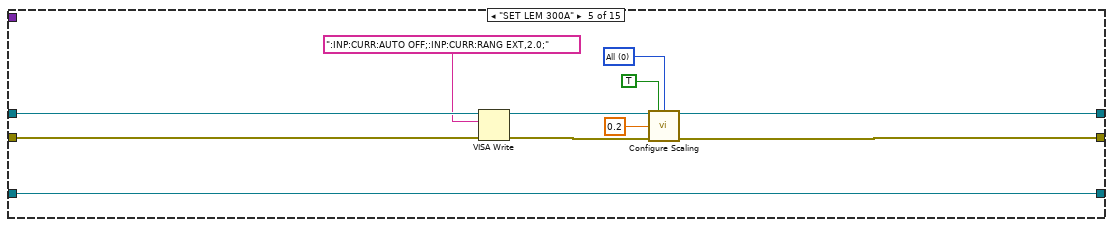
[diagram p14: hidden frame]
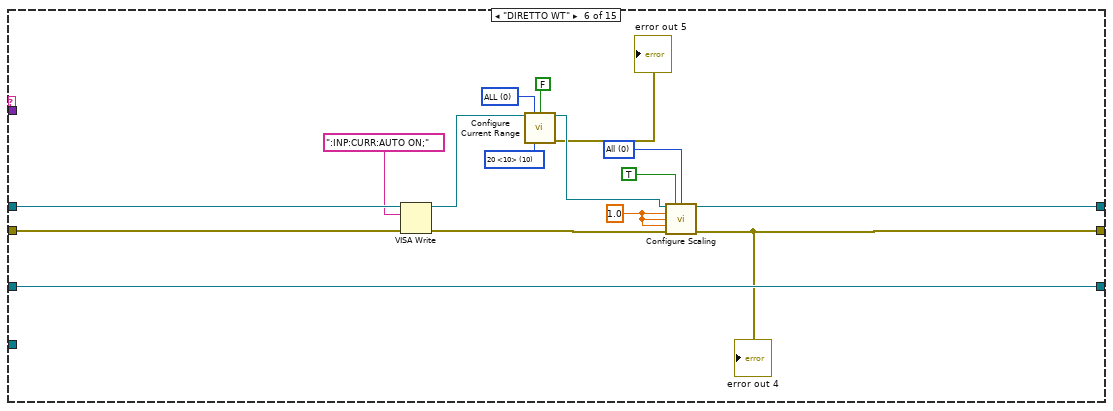
[diagram p15: hidden frame]
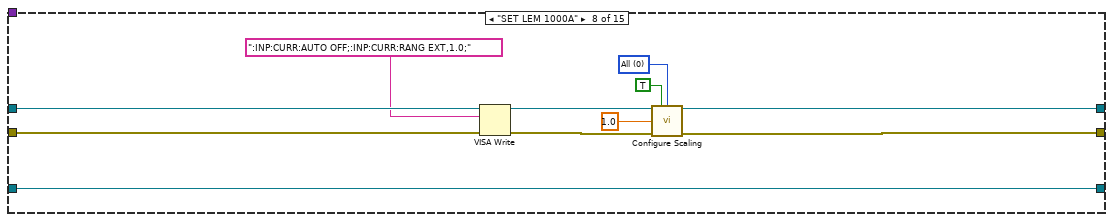
[diagram p16: hidden frame]
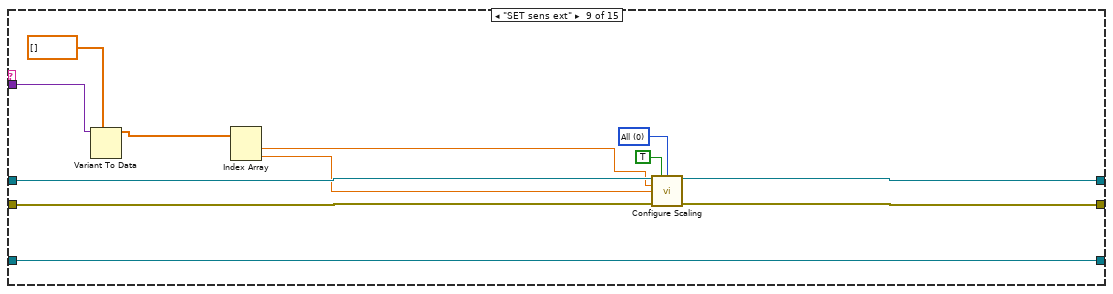
[diagram p17: hidden frame]
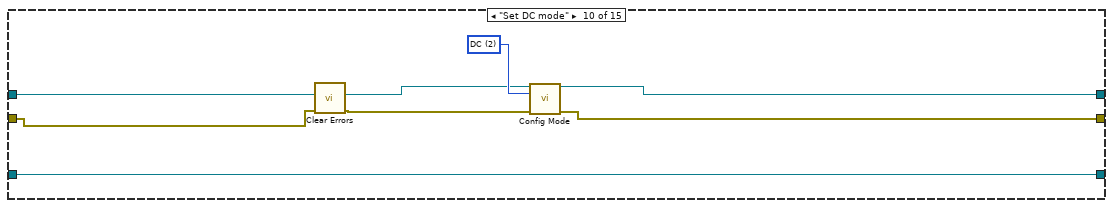
[diagram p18: hidden frame]
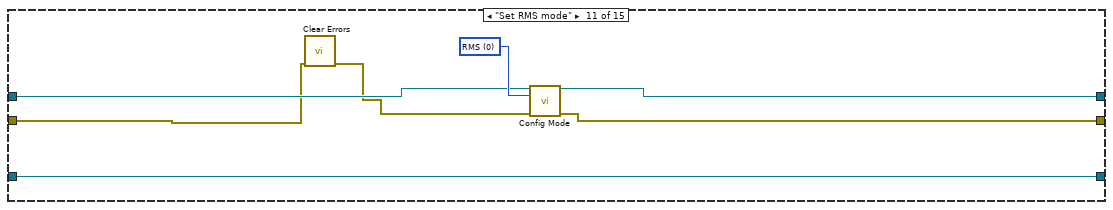
[diagram p19: hidden frame]
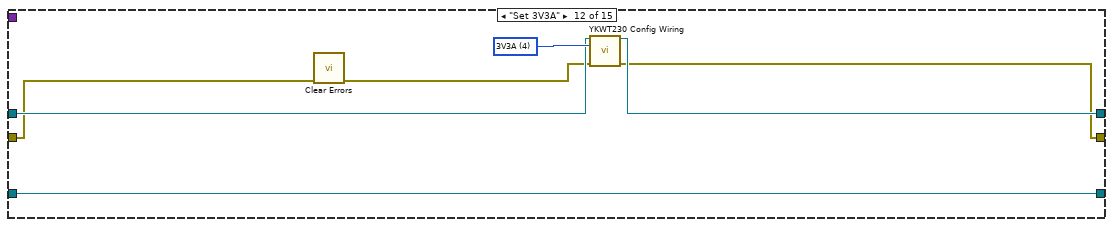
[diagram p20: hidden frame]
diagram:
  n1 = Obtain Queue(name (unnamed)="Queue Name", element data type=cluster{"String":string, "variant":variant} {"String"="", "variant"=variant} ("element")) -> (queue out=w6:refnum<queue>, error out=w5:errorcluster)  [unwired: 3 in, 1 out]
  n2 = Flush Queue(queue=w6, error in (no error)=w5) -> (queue out=w1:refnum<queue>, error out=w4:errorcluster)  [unwired: 1 out]
  n3 = Enqueue Element(queue=w1, element=cluster{"String":string, "variant":variant} {"String"="INITIALIZE", "variant"=variant}, error in (no error)=w4) -> (queue out=w13:refnum<queue>, error out=w12:errorcluster)  [unwired: 1 in, 1 out]
  n4 = while {
    shift-right: [w34] -> _
    shift-left: _ -> [w33]
    shift-right: [w31] -> w11
    shift-left: _ -> [w30]
    shift-right: [w28] -> w9
    shift-left: "error in (no error)" -> [w29]
    tunnel: w13 -> [w26]
    tunnel: w12 -> [w27]
    tunnel: [w18] -> w14
    tunnel: "simulazione" -> [w22]
    shift-right: [w21] -> _
    shift-left: _ -> [w20]
    i -> [w17]
    stop <- w18 stop-if-true
    # "PROCESSI CONTINUI"
    n5 = Dequeue Element(queue=w26, error in (no error)=w27) -> (queue out=w19:refnum<queue>, element=w25:cluster{"String":string, "variant":variant})  [unwired: 1 in, 2 out]
    n6 = call <userlib>:"loop timer.vi"("millisecond timer IN"=w33) -> ("millisecond timer OUT"=w34:u32, "LOOP TIME (ms)"=→"LOOP TIME (ms)":u32)  [unwired: 9 in]
    n7 = Unbundle(w25) -> ("String"=w24:string, "variant"=w23:variant)
    "STATO" <- w24
    n8 = case shown="\"SET LEM GENERICO\"" w24 {
      tunnel: [_ _ _ _ _ _ _ _ _ _ _ _ _ _ TRUE] -> w18
      tunnel: [w51 w81 w138 w182 w203 w219 w230 w241 w253 w260 w267 w274 w281 w283 w287] -> w31
      tunnel: w30 -> [_ w81 w138 w182 w203 w219 w230 w241 w253 w260 w267 w274 w281 w283 w287]
      tunnel: w29 -> [w48 w76 w137 w179 w201 w217 w228 w239 w248 w255 w262 w269 w276 w284 w286]
      tunnel: [w35 w70 w131 w180 w195 w212 w223 w232 w249 w256 w263 w270 w277 w284 w286] -> w28
      tunnel: w23 -> [_ _ _ w175 _ _ _ _ w246 _ _ _ _ _ _]
      tunnel: w22 -> [w46 w72 _ _ _ _ _ _ _ _ _ _ _ _ _]
      tunnel: [w37 w68 w132 w181 w197 w214 w225 w234 w250 w257 w264 w271 w278 w282 w285] -> w21
      tunnel: w20 -> [w45 w74 w136 w176 w202 w218 w229 w240 w247 w258 w265 w272 w279 w282 w285]
      tunnel: w19 -> [w43 w71 w133 _ _ _ _ _ _ _ _ _ _ _ _]
      frame "INITIALIZE", Default {
        w39 = u16 4 items=["", "1P3W", "3P3W", "3P4W", "3V3A"] ("Wiring (1: 1P3W)")
        w42 = u16 0 items=["RMS", "V-MEAN", "DC"] ("Mode (0: RMS)")
        (unwired) enum16{"INITIALIZE", "ENQUEUE", "STOP ALL"}."ENQUEUE" ("Function")
        # "CONFIGURE"
        n9 = case shown="False" w46 {
          tunnel: w48 -> [_ w67]
          tunnel: [w65 w67] -> w47
          tunnel: [w64 w66] -> w41
          tunnel: w45 -> [_ w66]
          frame False {
            n10 = call <vilib>:"Application Directory.vi"() -> ("Application Directory"=w58:path)
            n11 = Build Path(base path=w58, name or relative path="Settings\\WT330\\WT330_settings.txt") -> (appended path=w56:path)
            n12 = call-poly <vilib>:"Read From Spreadsheet File.vi"("delimiter (\\t)"="::" ("delimiter (\\t)"), "file path (dialog if empty)"=w56) -> ("all rows"=w54:string[][])  [unwired: 5 in, 4 out]
            n13 = Index Array(array=w54, index (col)=1 ("disabled index (col)")) -> (element=w52:string[])  [unwired: 1 in]
            n14 = Index Array(array=w52) -> (element=w61:string)  [unwired: 1 in]
            "VISA resource name" <- w61
            n15 = Concatenate Strings("TCPIP0::" ("string"), w61, "::INSTR" ("string")) -> (w60:string)
            n16 = call <instrlib>:"Initialize.vi"("Reset (True)"=FALSE, "VISA resource name"=w60) -> ("error out"=w65:errorcluster, "VISA resource name out"=w64:refnum<visa-resource-name>)  [unwired: 8 in]
          }
          frame True {
          }
        }
        n17 = call "SEND STATUS.vi"("ELEMENT"=DEVICE_NAME."WATTMETRO", "error in (no error)"=w47) -> ("error out"=w40:errorcluster)  [unwired: 9 in]
        n18 = Enqueue Element(queue=w43, element=cluster{"String":string, "variant":variant} {"String"="CONFIGURE", "variant"=variant}) -> ()  [unwired: 2 in, 3 out]
        n19 = control-ref of="This VI"() -> (w51:refnum<vi>)
        n20 = call <instrlib>:"Config Mode.vi"("VISA resource name"=w41, "Mode (0: RMS)"=w42, "error in (no error)"=w40) -> ("VISA resource name out"=w38:refnum<visa-resource-name>, "error out"=w36:errorcluster)  [unwired: 11 in]
        n21 = call <instrlib>:"YKWT230 Config Wiring.vi"("VISA resource name"=w38, "Wiring (1: 1P3W)"=w39, "error in (no error)"=w36) -> ("VISA resource name out"=w37:refnum<visa-resource-name>, "error out"=w35:errorcluster)  [unwired: 11 in]
        "Stopped" <- FALSE ("Stop")
      }
      frame "READ" {
        # "READ"
        n22 = case shown="False" w72 {
          tunnel: w76 -> [_ w115]
          tunnel: [w86 w115] -> w75
          tunnel: w74 -> [w105 w116]
          tunnel: [w104 w116] -> w68
          tunnel: [w89 w111] -> w73
          tunnel: [w86 _] -> w69
          frame False {
            (unwired) 4 ("index")
            n23 = call-poly <instrlib>:"Read Measurement.vi"("Number of Item (15)"="Number of Item (15)", "VISA resource name"=w105) -> ("error out"=w86:errorcluster, "Measurement"=w94:dbl[], "Function"=→"Function":string[], "VISA resource name out"=w104:refnum<visa-resource-name>)  [unwired: 6 in]
            "Measurement" <- w94
            n24 = Index Array(array=w94, index=30) -> (element=w102:dbl)
            n25 = global write "Globals.vi" "V SIGMA"(w102) -> ()
            n26 = Array Subset(array=w94, index=0, length=30) -> (w98:dbl[])
            n27 = Array Subset(array=w94, index=30, length=9) -> (w91:dbl[])
            n28 = Replace Array Subset(array=dbl[] [0.0, 0.0, 0.0, 0.0, 0.0, 0.0, 0.0, 0.0, 0.0, 0.0, 0.0, 0.0, 0.0, 0.0, 0.0, 0.0, 0.0, 0.0, 0.0, 0.0, 0.0, 0.0, 0.0, 0.0, 0.0, 0.0, 0.0, 0.0, 0.0, 0.0, 0.0, 0.0, 0.0, 0.0, 0.0, 0.0, 0.0, 0.0, 0.0, 0.0, 0.0, 0.0, 0.0, 0.0, 0.0, 0.0, 0.0, 0.0, 0.0, 0.0, 0.0, 0.0, 0.0, 0.0, 0.0, 0.0, 0.0, 0.0, 0.0, 0.0, 0.0, 0.0, 0.0, 0.0, 0.0, 0.0, 0.0, 0.0, 0.0, 0.0, 0.0, 0.0, 0.0, 0.0, 0.0, 0.0, 0.0, 0.0, 0.0, 0.0, 0.0, 0.0, 0.0, 0.0, 0.0, 0.0, 0.0, 0.0, 0.0, 0.0] ("Measure Value"), new element=w98, index=0) -> (w95:dbl[])
            n29 = Replace Array Subset(array=w95, new element=w91, index=60) -> (w90:dbl[])
            n30 = Array To Cluster(array=w90) -> (cluster=w89:T4)
          }
          frame True {
            n31 = global read "Global_All_Data.vi" "All Data"() -> (w113:T5)
            n32 = Unbundle By Name(w113) -> ("MISURE ALL.INTERFACCIA.AO non scalati.ALIM1 rif V"=w112:dbl, "MISURE ALL.INTERFACCIA.AO non scalati.ALIM1 rif F"=w110:dbl, "MISURE ALL.INTERFACCIA.DI (logici).ALIM 1 abilitato"=w109:bool, "MISURE ALL.INTERFACCIA.DI (logici).ALIM 1 run"=w108:bool, "MISURE ALL.INTERFACCIA.DI (logici).Start alimentazione AC"=w107:bool)
            n33 = Wait (ms)(milliseconds to wait=u32 200) -> ()  [unwired: 1 out]
            n34 = Compound Arithmetic op=AND(w109, w108, w107) -> (w106:bool)
            n35 = case shown="True" w106 {
              tunnel: w112 -> [_ w129]
              tunnel: [_ w128] -> w111
              tunnel: w110 -> [_ w127]
              frame False {
              }
              frame True {
                n36 = Random Number (0-1)() -> (number: 0 to 1=w125:dbl)
                n37 = Random Number (0-1)() -> (number: 0 to 1=w124:dbl)
                n38 = Divide(x=w124, y=3.0) -> (x/y=w122:dbl)
                n39 = Add(x=w125, y=w129) -> (x+y=w117:dbl)
                n40 = Add(x=w122, y=w127) -> (x+y=w126:dbl)
                n41 = local read "MISURE WT"() -> (w130:T1)
                n42 = Divide(x=w117, y=15.0) -> ()  [unwired: 1 out]
                n43 = Divide(x=w117, y=500.0) -> (x/y=w119:dbl)
                n44 = Bundle By Name(cluster=w130, "URMS 1"=w117, "URMS 2"=w117, "URMS 3"=w117, "F U 1"=w126, "F U 2"=w126, "F U 3"=w126, "URMS SIGMA"=w117, "IRMS SIGMA"="IRMS 3", "LAMBDA SIGMA"=w119, "IRMS 1"="IRMS 3", "IRMS 2"="IRMS 3", "IRMS 3"="IRMS 3") -> (w128:T1)
              }
            }
          }
        }
        "MISURE WT" <- w73
        n45 = case shown="No Error" w69 {
          tunnel: w71 -> [w82 w84]
          frame No Error {
            n46 = Enqueue Element(queue=w82, element=cluster{"String":string, "variant":variant} {"String"="READ", "variant"=variant}) -> ()  [unwired: 2 in, 3 out]
          }
          frame Error {
            n47 = Enqueue Element(queue=w84, element=cluster{"String":string, "variant":variant} {"String"="INITIALIZE", "variant"=variant}) -> ()  [unwired: 2 in, 3 out]
          }
        }
        n48 = Bundle By Name(cluster=T3 {"Array of elements"=[], "Single element"={"String"="READ WT", "variant"=variant}, "enque at\nopposite end (F)"=FALSE, "no replications (F)"=FALSE} ("Enqueue cluster"), "Single element.variant"=w73) -> (w77:T3)
        n49 = call <userlib>:"SMQ_MANAGER.vi"("Function"=enum16{"INITIALIZE", "ENQUEUE", "STOP ALL"}."ENQUEUE", "Queue name"="DATA_Q", "error in (no error)"=w75, "Enqueue cluster"=w77) -> ("error out"=w70:errorcluster)  [unwired: 7 in]
      }
      frame "CONFIGURE" {
        # "READ"
        n50 = case shown="False" TRUE {
          tunnel: w137 -> [w170 w171]
          tunnel: [w150 w171] -> w131
          tunnel: w136 -> [w169 w172]
          tunnel: [w151 w172] -> w132
          frame False {
            w143 = u8 255 items=["15 <7.5>"=8, "30 <15>"=15, "60 <30>"=30, "150 <75>"=75, "300 <150>"=150, "600 <300>"=255] ("Manual Range (600 <300> V)")
            w144 = 1 items=["Off", "On"] ("Set Filter (1: On)")
            w145 = u32 1 items=["Frequency", "Line"] ("Select Filter Type (0 : Frequency)")
            w149 = 3 items=["CF3"=3, "CF6"=6] ("Crest Factor (3: CF3)")
            w152 = 5 items=["1P2W"=1, "1P3W"=2, "3P3W"=3, "3P4W"=4, "3V3A"=5] ("Wiring A (1: 1p2W)")
            w157 = 1 items=["Off", "On"] ("Set Filter (1: On)")
            w158 = u32 0 items=["Frequency", "Line"] ("Select Filter Type (0 : Frequency)")
            n51 = call <vilib>:"Application Directory.vi"() -> ("Application Directory"=w167:path)
            n52 = Build Path(base path=w167, name or relative path="Settings\\WT330\\WT330_config.txt") -> (appended path=w165:path)
            n53 = call-poly <vilib>:"Read From Spreadsheet File.vi"("delimiter (\\t)"="::" ("delimiter (\\t)"), "file path (dialog if empty)"=w165) -> ("all rows"=w163:string[][])  [unwired: 5 in, 4 out]
            "WT330 Configuration" <- w163
            n54 = Index Array(array=w163, index (col)=1 ("disabled index (col)")) -> (element=w161:string[])  [unwired: 1 in]
            n55 = Fract/Exp String To Number(string=w161) -> (number=w160:dbl[])  [unwired: 3 in, 1 out]
            n56 = Index Array(array=w160) -> (element #1=w148:dbl, element #2=w159:dbl)  [unwired: 2 in]
            n57 = call <instrlib>:"Configure Scaling.vi"("VISA resource name"=w169, "Enable Scaling (T: Enable)"=TRUE, "VT Ratio (1.000)"=w148, "CT Ratio (1.000)"=w159, "error in (no error)"=w170) -> ("VISA resource name out"=w156:refnum<visa-resource-name>, "error out"=w155:errorcluster)  [unwired: 9 in]
            n58 = call <instrlib>:"Configure Wiring.vi"("VISA resource name"=w156, "Wiring A (1: 1p2W)"=w152, "error in (no error)"=w155) -> ("VISA resource name out"=w154:refnum<visa-resource-name>, "error out"=w153:errorcluster)  [unwired: 11 in]
            n59 = call <instrlib>:"Configure Filter.vi"("error in (no error)"=w153, "Set Filter (1: On)"=w157, "Select Filter Type (0 : Frequency)"=w158, "VISA resource name"=w154) -> ("error out"=w146:errorcluster, "VISA resource name out"=w147:refnum<visa-resource-name>)  [unwired: 6 in]
            n60 = call <instrlib>:"Configure Filter.vi"("error in (no error)"=w146, "Set Filter (1: On)"=w144, "Select Filter Type (0 : Frequency)"=w145, "VISA resource name"=w147) -> ("error out"=w140:errorcluster, "VISA resource name out"=w142:refnum<visa-resource-name>)  [unwired: 6 in]
            n61 = call <instrlib>:"Configure Voltage Range.vi"("VISA resource name"=w142, "error in (no error)"=w140, "Manual Range (600 <300> V)"=w143) -> ("VISA resource name out"=w141:refnum<visa-resource-name>, "error out"=w139:errorcluster)  [unwired: 11 in]
            n62 = call <instrlib>:"Configure Crest Factor Element.vi"("error in (no error)"=w139, "Crest Factor (3: CF3)"=w149, "VISA resource name"=w141) -> ("error out"=w150:errorcluster, "VISA resource name out"=w151:refnum<visa-resource-name>)  [unwired: 7 in]
          }
          frame True {
          }
        }
        n63 = Enqueue Element(queue=w133, element=cluster{"String":string, "variant":variant} {"String"="READ", "variant"=variant}) -> ()  [unwired: 2 in, 3 out]
      }
      frame "SET CT RATIO" {
        n64 = Variant To Data(error in=w179, type=0.0, Variant=w175) -> (data=w174:dbl, error out=w178:errorcluster)
        n65 = case shown="False" TRUE {
          tunnel: [w189 w192] -> w181
          tunnel: [w188 w191] -> w180
          tunnel: w178 -> [w186 w191]
          tunnel: w176 -> [w185 w192]
          tunnel: w174 -> [w184 _]
          frame False {
            n66 = call <instrlib>:"Configure Scaling.vi"("VISA resource name"=w185, "Enable Scaling (T: Enable)"=TRUE, "VT Ratio (1.000)"=1.0, "CT Ratio (1.000)"=w184, "Power Coefficient (1.000)"=1.0, "error in (no error)"=w186) -> ("VISA resource name out"=w189:refnum<visa-resource-name>, "error out"=w188:errorcluster)  [unwired: 8 in]
          }
          frame True {
          }
        }
      }
      frame "SET LEM 300A" {
        w200 = 0 items=["All", "1", "2", "3"] ("Element (0: All)")
        n67 = VISA Write ("VISA書き込み")(VISA resource name=w202, write buffer=":INP:CURR:AUTO OFF;:INP:CURR:RANG EXT,2.0;", error in (no error)=w201) -> (VISA resource name out=w198:refnum<visa-resource-name>, error out=w196:errorcluster)  [unwired: 1 out]
        n68 = call <instrlib>:"Configure Scaling.vi"("VISA resource name"=w198, "Enable Scaling (T: Enable)"=TRUE, "Element (0: All)"=w200, "CT Ratio (1.000)"=0.2, "error in (no error)"=w196) -> ("VISA resource name out"=w197:refnum<visa-resource-name>, "error out"=w195:errorcluster)  [unwired: 9 in]
      }
      frame "DIRETTO WT" {
        w204 = u8 10 items=["5m <2.5m>"=0, "10m <5m>"=0, "20m <10m>"=0, "50m <25m>"=0, "100m <50m>"=0, "200m <100m>"=0, "500m <250m>"=0, "1 <500m>"=0, "2 <1>"=1, "5 <2.5>"=2, "10 <5>"=5, "20 <10>"=10, "40 <20>"=20] ("Manual Range (20 <10> A)")
        w206 = u8 0 items=["ALL", "Custom"] ("Range Type (1: Custom)")
        w210 = 1.0 ("VT Ratio (1.000)")
        w216 = 0 items=["All", "1", "2", "3"] ("Element (0: All)")
        n69 = VISA Write ("VISA書き込み")(VISA resource name=w218, write buffer=":INP:CURR:AUTO ON;", error in (no error)=w217) -> (VISA resource name out=w209:refnum<visa-resource-name>, error out=w213:errorcluster)  [unwired: 1 out]
        n70 = call <instrlib>:"Configure Current Range.vi"("VISA resource name"=w209, "Range Type (1: Custom)"=w206, "Enable Auto Range (F: Disable)"=FALSE, "Manual Range (20 <10> A)"=w204) -> ("VISA resource name out"=w208:refnum<visa-resource-name>, "error out"=→"error out 5":errorcluster)  [unwired: 10 in]
        n71 = call <instrlib>:"Configure Scaling.vi"("VISA resource name"=w208, "Enable Scaling (T: Enable)"=TRUE, "Element (0: All)"=w216, "VT Ratio (1.000)"=w210, "CT Ratio (1.000)"=w210, "Power Coefficient (1.000)"=w210, "error in (no error)"=w213) -> ("VISA resource name out"=w214:refnum<visa-resource-name>, "error out"=w212:errorcluster)  [unwired: 7 in]
        "error out 4" <- w212
      }
      frame "SET LEM GENERICO" {
        w227 = 0 items=["All", "1", "2", "3"] ("Element (0: All)")
        n72 = VISA Write ("VISA書き込み")(VISA resource name=w229, write buffer="write buffer", error in (no error)=w228) -> (VISA resource name out=w220:refnum<visa-resource-name>, error out=w224:errorcluster)  [unwired: 1 out]
        n73 = call <instrlib>:"Configure Scaling.vi"("VISA resource name"=w220, "Enable Scaling (T: Enable)"=TRUE, "Element (0: All)"=w227, "CT Ratio (1.000)"="CT Ratio (1.000)", "error in (no error)"=w224) -> ("VISA resource name out"=w225:refnum<visa-resource-name>, "error out"=w223:errorcluster)  [unwired: 9 in]
        "error out 3" <- w223
      }
      frame "SET LEM 1000A" {
        w236 = 0 items=["All", "1", "2", "3"] ("Element (0: All)")
        n74 = VISA Write ("VISA書き込み")(VISA resource name=w240, write buffer=":INP:CURR:AUTO OFF;:INP:CURR:RANG EXT,1.0;", error in (no error)=w239) -> (VISA resource name out=w235:refnum<visa-resource-name>, error out=w233:errorcluster)  [unwired: 1 out]
        n75 = call <instrlib>:"Configure Scaling.vi"("VISA resource name"=w235, "Enable Scaling (T: Enable)"=TRUE, "Element (0: All)"=w236, "CT Ratio (1.000)"=1.0, "error in (no error)"=w233) -> ("VISA resource name out"=w234:refnum<visa-resource-name>, "error out"=w232:errorcluster)  [unwired: 9 in]
      }
      frame "SET sens ext" {
        w251 = 0 items=["All", "1", "2", "3"] ("Element (0: All)")
        n76 = Variant To Data(type=dbl[] [], Variant=w246) -> (data=w244:dbl[])  [unwired: 1 in, 1 out]
        n77 = Index Array(array=w244) -> (element #1=w243:dbl, element #2=w242:dbl)  [unwired: 2 in]
        n78 = call <instrlib>:"Configure Scaling.vi"("VISA resource name"=w247, "Enable Scaling (T: Enable)"=TRUE, "Element (0: All)"=w251, "VT Ratio (1.000)"=w243, "CT Ratio (1.000)"=w242, "error in (no error)"=w248) -> ("VISA resource name out"=w250:refnum<visa-resource-name>, "error out"=w249:errorcluster)  [unwired: 8 in]
      }
      frame "Set DC mode" {
        w259 = u16 2 items=["RMS", "V-MEAN", "DC"] ("Mode (0: RMS)")
        n79 = call <vilib>:"Clear Errors.vi"("error in (no error)"=w255) -> ("error out"=w254:errorcluster)  [unwired: 5 in, 1 out]
        n80 = call <instrlib>:"Config Mode.vi"("VISA resource name"=w258, "Mode (0: RMS)"=w259, "error in (no error)"=w254) -> ("VISA resource name out"=w257:refnum<visa-resource-name>, "error out"=w256:errorcluster)  [unwired: 11 in]
      }
      frame "Set RMS mode" {
        w266 = u16 0 items=["RMS", "V-MEAN", "DC"] ("Mode (0: RMS)")
        n81 = call <vilib>:"Clear Errors.vi"("error in (no error)"=w262) -> ("error out"=w261:errorcluster)  [unwired: 5 in, 1 out]
        n82 = call <instrlib>:"Config Mode.vi"("VISA resource name"=w265, "Mode (0: RMS)"=w266, "error in (no error)"=w261) -> ("VISA resource name out"=w264:refnum<visa-resource-name>, "error out"=w263:errorcluster)  [unwired: 11 in]
      }
      frame "Set 3V3A" {
        w273 = u16 4 items=["", "1P3W", "3P3W", "3P4W", "3V3A"] ("Wiring (1: 1P3W)")
        n83 = call <vilib>:"Clear Errors.vi"("error in (no error)"=w269) -> ("error out"=w268:errorcluster)  [unwired: 5 in, 1 out]
        n84 = call <instrlib>:"YKWT230 Config Wiring.vi"("VISA resource name"=w272, "Wiring (1: 1P3W)"=w273, "error in (no error)"=w268) -> ("VISA resource name out"=w271:refnum<visa-resource-name>, "error out"=w270:errorcluster)  [unwired: 11 in]
      }
      frame "Set 3P4W" {
        w280 = u16 3 items=["", "1P3W", "3P3W", "3P4W", "3V3A"] ("Wiring (1: 1P3W)")
        n85 = call <vilib>:"Clear Errors.vi"("error in (no error)"=w276) -> ("error out"=w275:errorcluster)  [unwired: 5 in, 1 out]
        n86 = call <instrlib>:"YKWT230 Config Wiring.vi"("VISA resource name"=w279, "Wiring (1: 1P3W)"=w280, "error in (no error)"=w275) -> ("VISA resource name out"=w278:refnum<visa-resource-name>, "error out"=w277:errorcluster)  [unwired: 11 in]
      }
      frame "OPEN" {
        n87 = call <userlib>:"easy open VI panel.vi"("VI in"=w283) -> ()  [unwired: 10 in, 1 out]
      }
      frame "STOP" {
      }
    }
    "Numeric" <- w17
  }
  n88 = while {
    tunnel: w1 -> [w289]
    stop <- w290 stop-if-true
    # "PROCESSI A EVENTI"
    n89 = event shown="[3] \"DIRETTO WT\": Value Change" {
      selector: _ -> [_ _ _ _ _ _ _]
      dyn-events: _ -> [_ _ _ _ _ _ _]
      timeout: _ -> [_ _ _ _ _ _ _]
      tunnel: [w291 _ _ _ _ _ _] -> w290
      tunnel: w289 -> [_ w292 w294 w296 w298 w300 w302]
      event "Stopped": Value Change {
        n90 = event-data() -> ("NewVal"=w291:bool)  [unwired: 1 in]
      }
      event "LEM 300": Value Change {
        n91 = event-data() -> ()  [unwired: 1 in, 6 out]
        n92 = Enqueue Element(queue=w292, element=cluster{"String":string, "variant":variant} {"String"="SET LEM 300A", "variant"=variant}) -> ()  [unwired: 2 in, 3 out]
      }
      event "LEM GENERICO": Value Change {
        n93 = event-data() -> ()  [unwired: 1 in, 6 out]
        n94 = Enqueue Element(queue=w294, element=cluster{"String":string, "variant":variant} {"String"="SET LEM GENERICO", "variant"=variant}) -> ()  [unwired: 2 in, 3 out]
      }
      event "DIRETTO WT": Value Change {
        n95 = event-data() -> ()  [unwired: 1 in, 6 out]
        n96 = Enqueue Element(queue=w296, element=cluster{"String":string, "variant":variant} {"String"="DIRETTO WT", "variant"=variant}) -> ()  [unwired: 2 in, 3 out]
      }
      event "LEM 1000": Value Change {
        n97 = event-data() -> ()  [unwired: 1 in, 6 out]
        n98 = Enqueue Element(queue=w298, element=cluster{"String":string, "variant":variant} {"String"="SET LEM 1000A", "variant"=variant}) -> ()  [unwired: 2 in, 3 out]
      }
      event "dc mode": Value Change {
        n99 = event-data() -> ()  [unwired: 1 in, 6 out]
        n100 = Enqueue Element(queue=w300, element=cluster{"String":string, "variant":variant} {"String"="Set DC mode", "variant"=variant}) -> ()  [unwired: 2 in, 3 out]
      }
      event "rms mode": Value Change {
        n101 = event-data() -> ()  [unwired: 1 in, 6 out]
        n102 = Enqueue Element(queue=w302, element=cluster{"String":string, "variant":variant} {"String"="Set RMS mode", "variant"=variant}) -> ()  [unwired: 2 in, 3 out]
      }
    }
  }
  n103 = disable-structure shown="Enabled" {
    disable-tunnel: [w304 _] -> _
    frame Disabled {
      n104 = for {
        tunnel: "Measurement 2" -> [w312] mode=indexing
        tunnel: [w306] -> w304 mode=indexing
        n105 = Random Number (0-1)() -> (number: 0 to 1=w310:dbl)
        n106 = Divide(x=w310, y=100.0) -> (x/y=w308:dbl)
        n107 = Add(x=w308, y=0.995) -> (x+y=w307:dbl)
        n108 = Multiply(x=w307, y=w312) -> (x*y=w306:dbl)
      }
    }
    frame Enabled {
    }
  }
  n109 = property on="Stopped" class="Bool (strict)"("Val(Sgnl)"=w14) -> ()  [unwired: 2 in, 2 out]
  n110 = call "SEND STATUS.vi"("ELEMENT"=DEVICE_NAME."WATTMETRO", "error in (no error)"=w9) -> ("error out"=w8:errorcluster)  [unwired: 9 in]
  n111 = flat-sequence {
    tunnel: w11 -> [w318]
    tunnel: w8 -> [w313]
    frame #0 {
      n112 = property class="VI"(reference=w318) -> (reference out=w314:refnum<vi>, "FP.State"=w317:T31)  [unwired: 1 in, 1 out]
      n113 = Not Equal?(x=T31."Closed", y=w317) -> (x != y?=w315:bool)
      n114 = case shown="True" w315 {
        tunnel: w314 -> [_ w319]
        frame False {
        }
        frame True {
          n115 = invoke class="VI" method="FP.Close"(reference=w319) -> ()  [unwired: 2 in, 3 out]
        }
      }
      "error out" <- w313
    }
  }
